vi "Autopatch-v2.2_systemauto.vi"() -> ()   [LabVIEW 2018]
uses:
  <vilib>/userdefined/High Color/IMAQdx.ctl
  <vilib>/DAQmx/write.llb/DAQmx Write (Analog DBL 1Chan 1Samp).vi
  <vilib>/DAQmx/write.llb/DAQmx Write (Analog Wfm 1Chan NSamp).vi
  <vilib>/DAQmx/read.llb/DAQmx Read (Analog Wfm 1Chan NSamp).vi
  <vilib>/Analysis/baseanly.llb/Mean (DBL).vi
  <vilib>/DAQmx/create/channels.llb/DAQmx Create Channel (AO-Voltage-Basic).vi
  <vilib>/DAQmx/miscellaneous.llb/DAQmx Fill In Error Info.vi
  <vilib>/DAQmx/create/channels.llb/DAQmx Create Channel (AI-Voltage-Basic).vi
  <vilib>/DAQmx/configure/timing.llb/DAQmx Timing (Sample Clock).vi
  <vilib>/DAQmx/configure/trigger.llb/DAQmx Start Trigger (Digital Edge).vi
  <vilib>/Waveform/WDTOps.llb/WDT Waveform Duration DBL.vi
  <vilib>/addons/control/pid/pid.llb/PID (DBL).vi
  <vilib>/vision/driver/NI_Vision_Acquisition_Software.lvlib
  <resource>/objmgr/daqmx.rc
  <vilib>/Analysis/NI_AALBase.lvlib
  <vilib>/measure/NI_MABase.lvlib
  <vilib>/vision/NI_Vision_Development_Module.lvlib
  <vilib>/addons/control/pid/NI_PID_pid.lvlib
  <vilib>/Analysis/NI_AALPro.lvlib
panel:
  out "最大值":dbl
  out "Matches 2":T1(array[cluster]) {"Bounding Box"."y" format="%.2f"; "Bounding Box"."x" format="%.2f"; "Position"."y" format="%.2f"; "Position"."x" format="%.2f"; "Score" format="%.2f"; "Scale" format="%.2f"; "Angle" format="%.2f"}
  in  "基路径40":path=path "D:/韩宇/程序/CCD/模板40倍.jpg"
  out "Particle Measurements (Pixels) 2":dbl[][](array[numeric]) format="%.2f"
  in  "Pixel Measurements 2":T2[](array[typedef])=[2] items=["Center of Mass X", "Center of Mass Y", "First Pixel X", "First Pixel Y", "Bounding Rect Left", "Bounding Rect Top", "Bounding Rect Right", "Bounding Rect Bottom", "Max Feret Diameter Start X", "Max Feret Diameter Start Y", "Max Feret Diameter End X", "Max Feret Diameter End Y", "Max Horiz. Segment Length Left", "Max Horiz. Segment Length Right", "Max Horiz. Segment Length Row", "-", "Bounding Rect Width", "Bounding Rect Height", "Bounding Rect Diagonal", "Perimeter", "Convex Hull Perimeter", "Holes' Perimeter", "Max Feret Diameter", "Equivalent Ellipse Major Axis", "Equivalent Ellipse Minor Axis", "Equivalent Ellipse Minor Axis (Feret)", "Equivalent Rect Long Side", "Equivalent Rect Short Side", "Equivalent Rect Diagonal", "Equivalent Rect Short Side (Feret)", "Average Horiz. Segment Length", "Average Vert. Segment Length", "Hydraulic Radius", "Waddel Disk Diameter", "-", "Area", "Holes' Area", "Particle & Holes' Area", "Convex Hull Area", "Image Area", "-", "Number of Holes", "Number of Horiz. Segments", "Number of Vert. Segments", "-", "Orientation", "Max Feret Diameter Orientation", "-", "% Area/Image Area", "% Area/(Particle & Holes' Area)", "Ratio of Equivalent Ellipse Axes", "Ratio of Equivalent Rect Sides", "-", "Elongation Factor", "Compactness Factor", "Heywood Circularity Factor", "Type Factor", "-", "Sum X", "Sum Y", "Sum XX", "Sum XY", "Sum YY", "Sum XXX", "Sum XXY", "Sum XYY", "Sum YYY", "-", "Moment of Inertia XX", "Moment of Inertia XY", "Moment of Inertia YY", "Moment of Inertia XXX", "Moment of Inertia XXY", "Moment of Inertia XYY", "Moment of Inertia YYY", "Norm. Moment of Inertia XX", "Norm. Moment of Inertia XY", "Norm. Moment of Inertia YY", "Norm. Moment of Inertia XXX", "Norm. Moment of Inertia XXY", "Norm. Moment of Inertia XYY", "Norm. Moment of Inertia YYY", "Hu Moment 1", "Hu Moment 2", "Hu Moment 3", "Hu Moment 4", "Hu Moment 5", "Hu Moment 6", "Hu Moment 7"]
  out "傅里叶最大值":dbl
  out "傅里叶数组":bool[](array[boolean])
  in  "傅里叶状态机":u16(ring) items=["傅里叶初始", "傅里叶循环", "傅里叶暂停", "傅里叶结束"]
  out "图像检测到":bool=TRUE
  out "自动封接开始时间":u32
  out "针下降次数":i32
  in  "自动测试":bool
  in  "图像网络检测":bool
  out "写入的字节":i32
  out "数据输出 3":string
  out "X 3":i32
  out "Y 3":i32
  out "error IO":errorcluster
  out "裁剪数组":i32[](array[numeric])
  out "Y 2":i32
  out "X 2":i32
  in  "针尖自动移动 2":bool
  in  "升Z轴找针":bool
  out "已发送图像":bool
  in  "傅里叶":bool
  in  "自动对焦状态机":u16(ring) items=["自动对焦初始", "自动对焦循环", "自动对焦结束"]
  in  "自动扫描状态机":u16(ring) items=["自动扫描初始", "自动扫描循环", "自动扫描结束"]
  out "startY":dbl
  in  "手动暂停":bool
  out "Particle Measurements (Pixels)":dbl[][](array[numeric]) format="%.2f"
  in  "Pixel Measurements":T2[](array[typedef])=[3] items=["Center of Mass X", "Center of Mass Y", "First Pixel X", "First Pixel Y", "Bounding Rect Left", "Bounding Rect Top", "Bounding Rect Right", "Bounding Rect Bottom", "Max Feret Diameter Start X", "Max Feret Diameter Start Y", "Max Feret Diameter End X", "Max Feret Diameter End Y", "Max Horiz. Segment Length Left", "Max Horiz. Segment Length Right", "Max Horiz. Segment Length Row", "-", "Bounding Rect Width", "Bounding Rect Height", "Bounding Rect Diagonal", "Perimeter", "Convex Hull Perimeter", "Holes' Perimeter", "Max Feret Diameter", "Equivalent Ellipse Major Axis", "Equivalent Ellipse Minor Axis", "Equivalent Ellipse Minor Axis (Feret)", "Equivalent Rect Long Side", "Equivalent Rect Short Side", "Equivalent Rect Diagonal", "Equivalent Rect Short Side (Feret)", "Average Horiz. Segment Length", "Average Vert. Segment Length", "Hydraulic Radius", "Waddel Disk Diameter", "-", "Area", "Holes' Area", "Particle & Holes' Area", "Convex Hull Area", "Image Area", "-", "Number of Holes", "Number of Horiz. Segments", "Number of Vert. Segments", "-", "Orientation", "Max Feret Diameter Orientation", "-", "% Area/Image Area", "% Area/(Particle & Holes' Area)", "Ratio of Equivalent Ellipse Axes", "Ratio of Equivalent Rect Sides", "-", "Elongation Factor", "Compactness Factor", "Heywood Circularity Factor", "Type Factor", "-", "Sum X", "Sum Y", "Sum XX", "Sum XY", "Sum YY", "Sum XXX", "Sum XXY", "Sum XYY", "Sum YYY", "-", "Moment of Inertia XX", "Moment of Inertia XY", "Moment of Inertia YY", "Moment of Inertia XXX", "Moment of Inertia XXY", "Moment of Inertia XYY", "Moment of Inertia YYY", "Norm. Moment of Inertia XX", "Norm. Moment of Inertia XY", "Norm. Moment of Inertia YY", "Norm. Moment of Inertia XXX", "Norm. Moment of Inertia XXY", "Norm. Moment of Inertia XYY", "Norm. Moment of Inertia YYY", "Hu Moment 1", "Hu Moment 2", "Hu Moment 3", "Hu Moment 4", "Hu Moment 5", "Hu Moment 6", "Hu Moment 7"]
  in  "手动换物镜":bool
  out "扫描变量":dbl=10.0
  in  "自动扫描":bool
  in  "自动移至工作位置":bool
  out "Z":dbl
  out "Y":dbl
  out "X":dbl
  out "自动接触初始":i32
  in  "枚举":enum16{"200ms", "500ms", "1000ms", ""}(ring)
  out "dX/dt":dbl[](array[numeric])
  in  "下降/向右":bool
  in  "down":bool
  in  "up":bool
  out "Z轴坐标":string
  in  "调焦步伐/um":i64(ring)=3 items=["1", "10", "100", "1000", "10000"]
  in  "停止运动":bool
  in  "设置移动步长":bool
  in  "返回Z轴坐标":bool
  out "x*y":dbl
  out "电阻值":dbl
  in  "钳制电位":i16(ring) items=["0mv", "-70mv"]
  out "起始破膜时间":u32
  in  "自动破膜":bool
  in  "控制箱刺激ON\n/放大器刺激":bool=TRUE
  in  "自动封接":bool
  in  "保存数据":bool
  out "是否匹配到？":bool
  in  "PID gains":T3={"proportional gain (Kc)"=-0.05, "integral time (Ti, min)"=0.0, "derivative time (Td, min)"=0.0} caption="PID增益" {"derivative time (Td, min)" format="%.3f"; "integral time (Ti, min)" format="%.3f"; "proportional gain (Kc)" format="%.3f"}
  in  "PID gains 2":T3={"proportional gain (Kc)"=0.05, "integral time (Ti, min)"=0.0, "derivative time (Td, min)"=0.0} caption="PID增益" {"derivative time (Td, min)" format="%.3f"; "integral time (Ti, min)" format="%.3f"; "proportional gain (Kc)" format="%.3f"}
  out "x+y 2":i16
  out "调焦值2":dbl
  out "调焦值3":dbl
  out "调焦值4":dbl
  out "对焦变量":dbl
  in  "聚焦值数组":dbl[](array[numeric])
  in  "下降步伐/um":dbl=1.0
  in  "自动接触":bool
  out "清晰度评价函数":dbl(graph)
  in  "针尖自动移动":bool
  in  "针尖细对焦":bool
  in  "针尖粗对焦":bool
  out "二值化":T4(plugin-control)
  in  "Range":cluster{"Lower value":sgl, "Upper value":sgl}={"Lower value"=0.0, "Upper value"=157.0} {"Upper value" format="%.2f"; "Lower value" format="%.2f"}
  in  "Operation":T5(ring)=enum."Dilate"
  in  "Number of Erosion":i32=10
  out "Right":dbl
  out "目标坐标":i32[](array[numeric])
  in  "针尖模板匹配":bool=TRUE
  in  "基路径20":path=path "D:/韩宇/程序/CCD/针尖水下模板20X.jpg"
  out "Number of Matches":i32
  in  "Minimum Contrast":i32 min=0 max=255 step=1
  in  "Minimum Match Score":sgl=650.0 min=0 max=1000 format="%.2f"
  in  "Number of Matches Requested":i32=1 min=1
  in  "Match Mode":u16(ring) items=["Shift Invariant", "Rotation Invariant"]
  out "针尖坐标":sgl[](array[numeric])
  in  "入液阻值校准":bool
  out "校准的入液阻值":dbl
  out "错误输出 3":errorcluster caption="错误输出"
  in  "低负开关":bool
  in  "低正开关":bool
  in  "大气压":bool
  in  "高负开关":bool
  in  "高正开关":bool
  in  "case":dbl
  out "测量值":dbl
  out "给定值":dbl
  out "输出气压波形图表":cluster{dbl, "低负":dbl}(graph)
  in  "低负":sgl(knob)=-0.45548448
  in  "高负":sgl(knob)=-5.0
  in  "低正":sgl(knob)=0.49642125 scale=0.0..2.0
  in  "高正":sgl(knob)=10.718505 scale=0.0..15.0
  in  "采样率":u32=255
  in  "DevIndex":i32
  in  "Holding Voltage":dbl=-70.0
  out "Negative Peak":dbl
  out "阻值波形图表":dbl(graph)
  out "Resistance(MΩ)":dbl
  out "！":bool
  in  "电压钳/电流钳":u16(ring) items=["Voltage Clamp", "Current Clamp"]
  out "电流信号波形图":waveform(dbl)(graph)
  in  "frequency":dbl=20.0
  in  "Averaging":i32=5
  in  "amplitude":dbl=0.01
  in  "阻值数组":dbl[](array[numeric])
  out "循环时间":u32
  out "Image":T4(plugin-control)
  out "错误输出":errorcluster
  in  "停止":bool
  in  "Session In":T6="cam1"
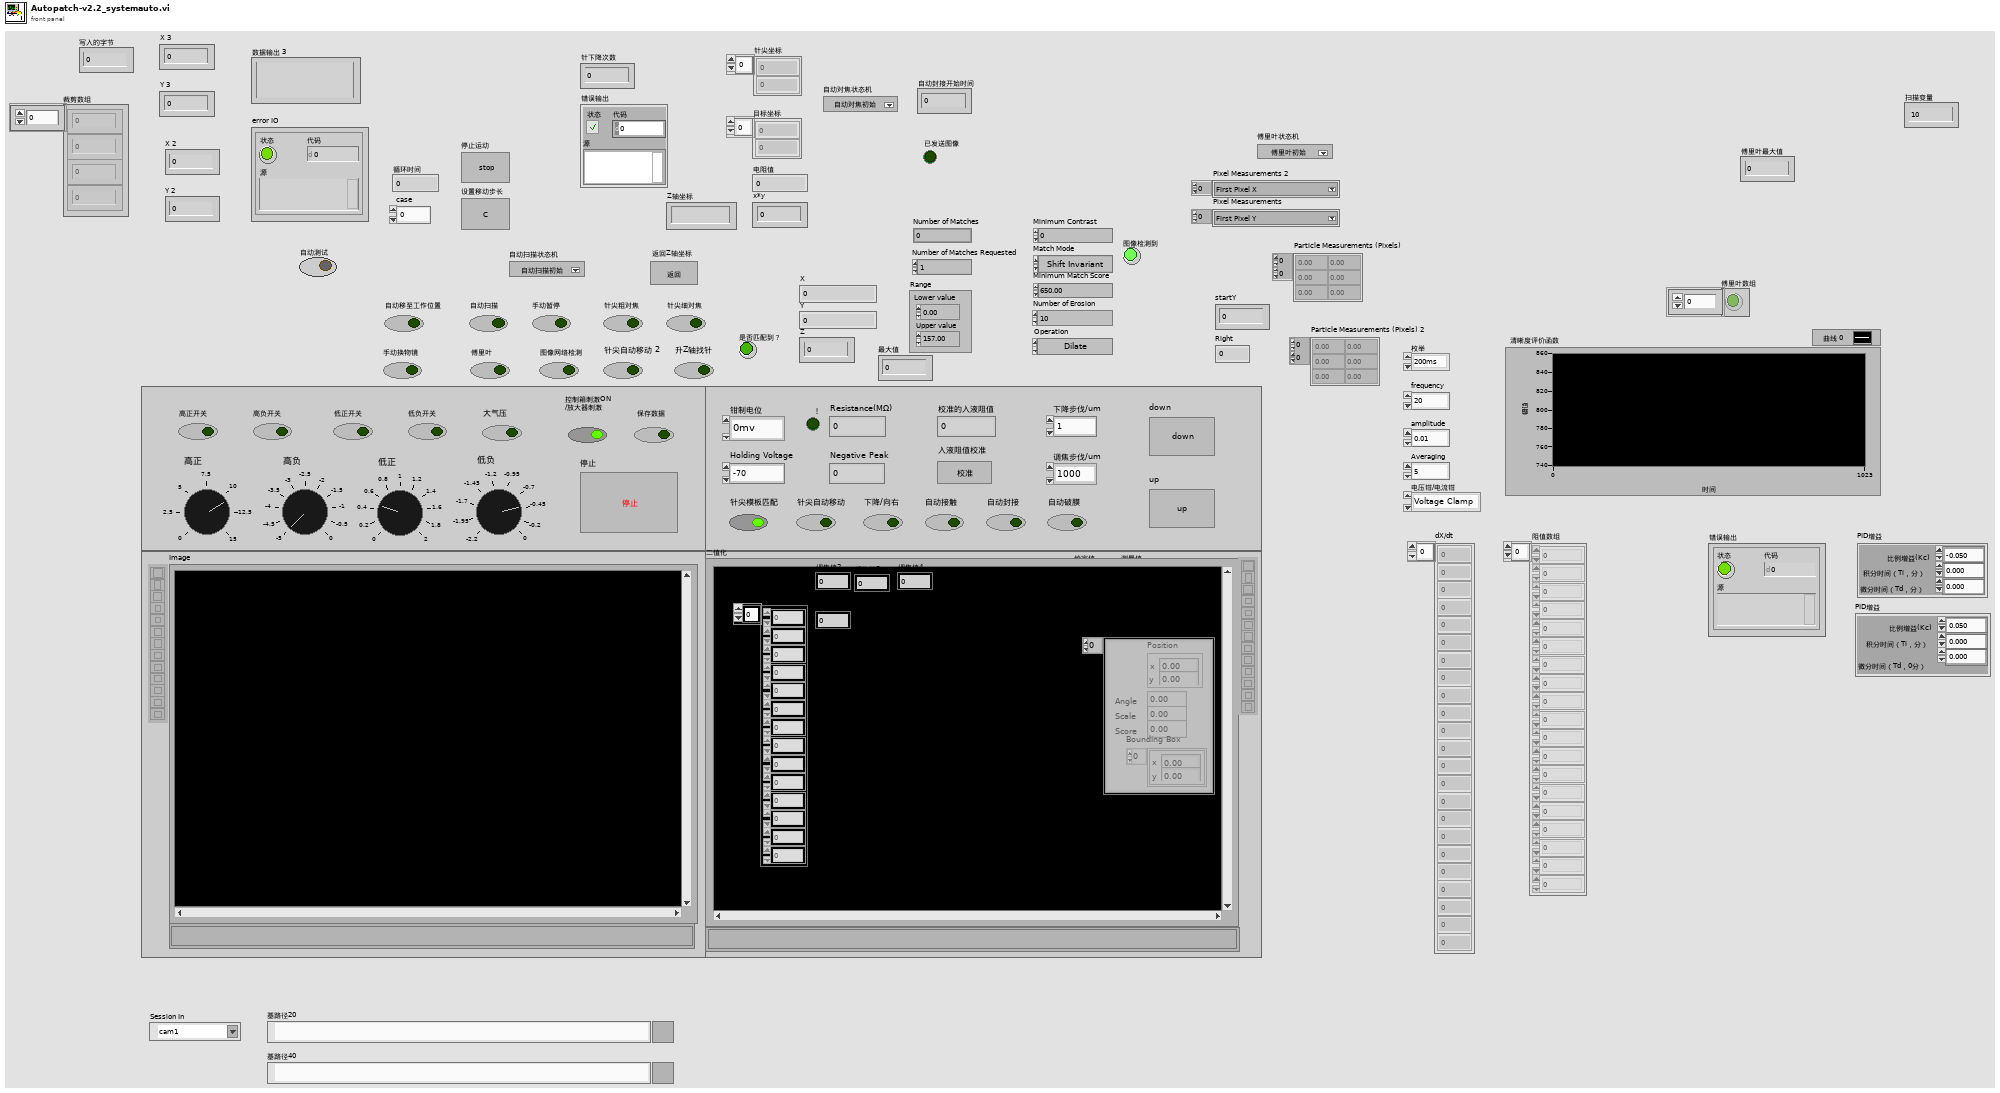
[diagram p1: front panel]
types:
  T1 = cluster{"Position":cluster{"x":sgl, "y":sgl}, "Angle":sgl, "Scale":sgl, "Score":sgl, "Bounding Box":cluster{"x":sgl, "y":sgl}[]}[]
  T2 = typedef "Particle Parameters" = i32
  T3 = cluster{"proportional gain (Kc)":dbl, "integral time (Ti, min)":dbl, "derivative time (Td, min)":dbl}
  T4 = typedef "IMAQ Image.ctl" = refnum<image>
  T5 = enum32{"AutoM", "Close", "Dilate", "Erode", "Gradient", "Gradient out", "Gradient in", "Hit miss", "Open", "PClose", "POpen", "Thick", "Thin"}
  T6 = typedef "IMAQdx.ctl" = refnum<k21>
  T7 = typedef "Image Type" = u32
  T8 = enum16{"open", "replace", "create", "open or create", "replace or create", "replace or create with confirmation"}
  T9 = cluster{"Averaging":i32, "frequency":dbl, "amplitude":dbl, "Proportion":dbl, "Fs":dbl}
  T10 = enum16{"Sine Wave", "Triangle Wave", "Square Wave", "Sawtooth Wave"}
  T11 = cluster{"Global Rectangle":i32[], "Contours":cluster{"Contour Type":u32, "ROI Type":u32, "Points":i32[]}[]}
  T12 = cluster{"Position":cluster{"x":sgl, "y":sgl}, "Angle":sgl, "Scale":sgl, "Score":sgl, "Bounding Box":cluster{"x":sgl, "y":sgl}[]}
  T13 = enum32{"Real", "Imaginary", "Magnitude", "Phase"}
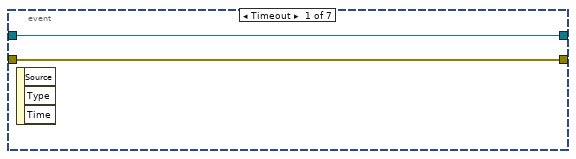
[diagram p3: hidden frame]
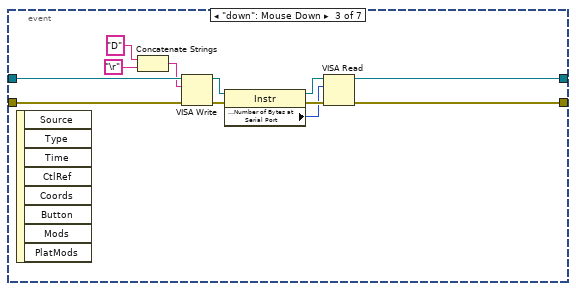
[diagram p4: hidden frame]
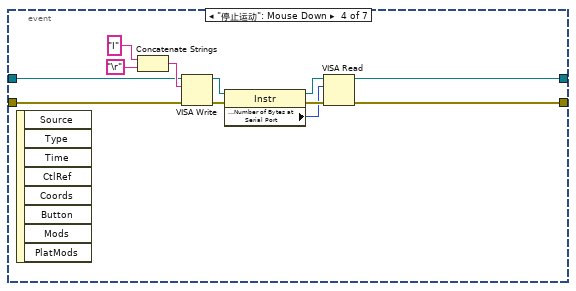
[diagram p5: hidden frame]
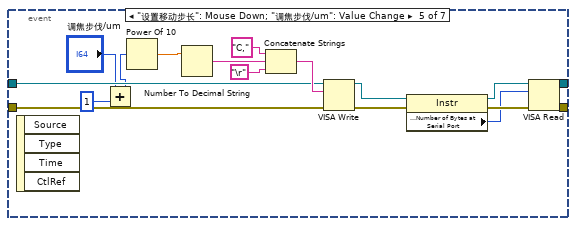
[diagram p6: hidden frame]
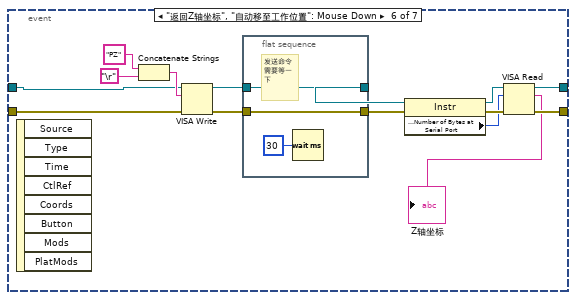
[diagram p7: hidden frame]
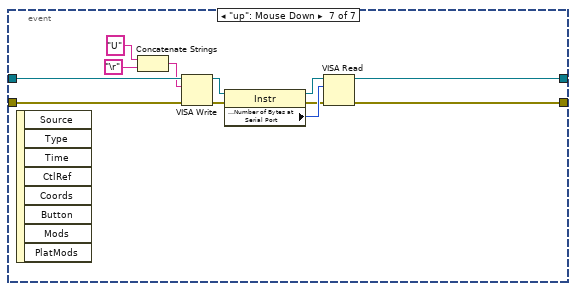
[diagram p8: hidden frame]
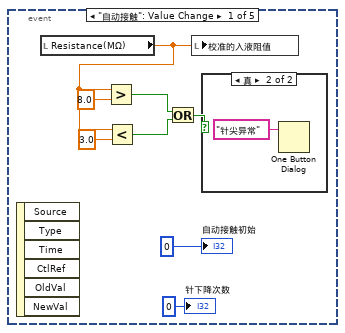
[diagram p9: hidden frame]
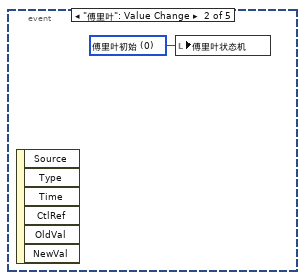
[diagram p11: hidden frame]
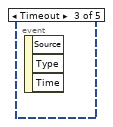
[diagram p12: hidden frame]
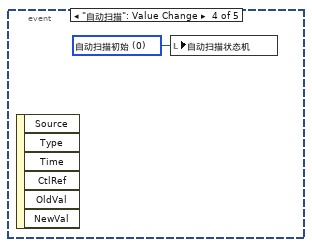
[diagram p13: hidden frame]
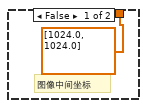
[diagram p14: hidden frame]
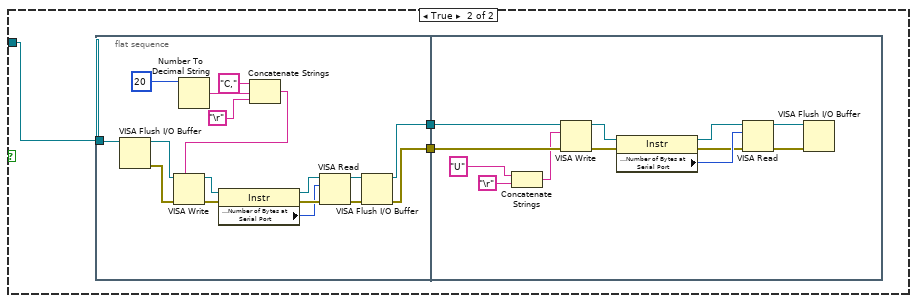
[diagram p16: hidden frame]
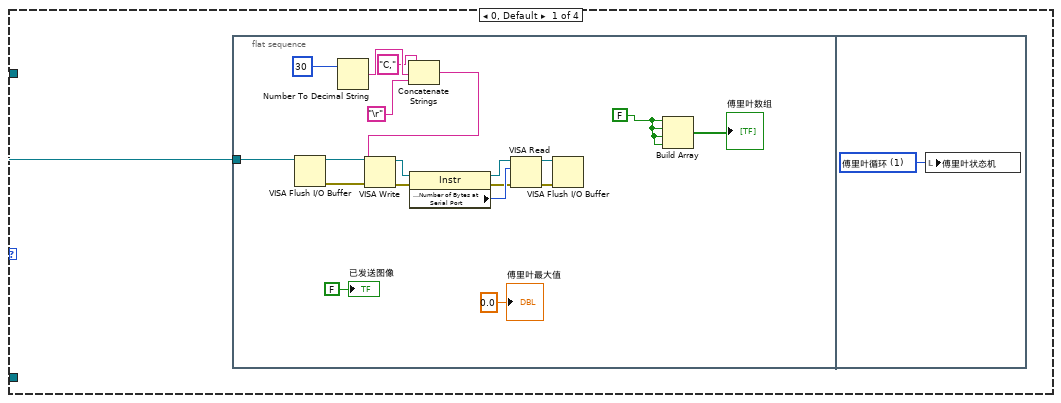
[diagram p18: hidden frame]
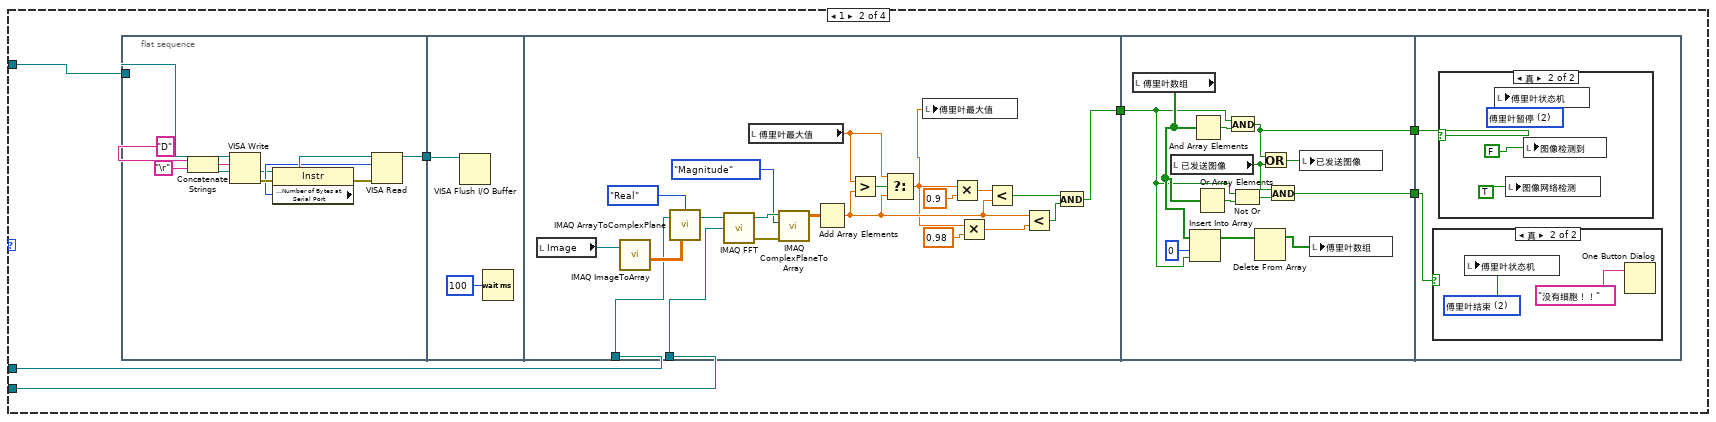
[diagram p19: hidden frame]
diagram:
  w5 = T7 0 items=["Grayscale (U8)", "Grayscale (I16)", "Grayscale (SGL)", "Complex (CSG)", "RGB (U32)", "HSL (U32)", "RGB (U64)", "Grayscale (U16)"] ("Image Type")
  w16 = T7 3 items=["Grayscale (U8)", "Grayscale (I16)", "Grayscale (SGL)", "Complex (CSG)", "RGB (U32)", "HSL (U32)", "RGB (U64)", "Grayscale (U16)"] ("Image Type")
  w14 = T7 3 items=["Grayscale (U8)", "Grayscale (I16)", "Grayscale (SGL)", "Complex (CSG)", "RGB (U32)", "HSL (U32)", "RGB (U64)", "Grayscale (U16)"] ("Image Type")
  w68 = T7 0 items=["Grayscale (U8)", "Grayscale (I16)", "Grayscale (SGL)", "Complex (CSG)", "RGB (U32)", "HSL (U32)", "RGB (U64)", "Grayscale (U16)"] ("Image Type")
  w82 = FALSE
  # "XY移动平台"
  # "Mp285"
  # "保存数据"
  n1 = case shown="真" "自动测试" {
    frame False {
    }
    frame True {
      n2 = flat-sequence {
        frame #0 {
          n3 = One Button Dialog(message="请安装玻璃电极并手动更换20倍显微镜" ("消息")) -> ()  [unwired: 1 in, 1 out]
        }
        frame #1 {
          n4 = local write "针尖粗对焦"(FALSE ("针尖粗对焦")) -> ()
          n5 = local write "针尖细对焦"(FALSE ("针尖细对焦")) -> ()
          n6 = local write "自动移至工作位置"(TRUE ("自动移至工作位置")) -> ()
          n7 = local write "傅里叶"(FALSE ("傅里叶")) -> ()
          n8 = local write "针尖自动移动"(FALSE ("针尖自动移动")) -> ()
          n9 = local write "针尖自动移动 2"(FALSE ("针尖自动移动 2")) -> ()
          n10 = local write "自动扫描"(FALSE ("自动扫描")) -> ()
          n11 = local write "手动换物镜"(FALSE ("手动换物镜")) -> ()
          n12 = local write "自动接触"(FALSE ("自动接触")) -> ()
          n13 = local write "升Z轴找针"(FALSE ("升Z轴找针")) -> ()
        }
      }
    }
  }
  n14 = flat-sequence {
    tunnel: [w156] -> w129
    frame #0 {
      # "选择刺激方式，内部刺激更准"
      n15 = Array Size(array="阻值数组") -> (size(s)=w155:i32)
      n16 = Delete From Array(array="阻值数组", length=w155) -> (array with subset deleted=w153:dbl[])  [unwired: 1 in, 1 out]
      n17 = local write "阻值数组"(w153) -> ()
    }
    frame #1 {
      # "波形个数"
      # "计算电阻波形比例"
      n18 = Bundle("Averaging"="Averaging", "frequency"="frequency", "amplitude"="amplitude", "Proportion"=0.4, "Fs"=20000.0) -> (w156:T9)  [unwired: 1 in]
    }
  }
  n19 = call "OpenDevice.vi"("DevIndex"="DevIndex") -> ("错误输出"=w109:errorcluster, "DevIndex Output"=w107:i32)  [unwired: 9 in]
  n20 = call "SetUSB2AiRange.vi"("错误输入（无错误）"=w109, "Range"=sgl 5.0, "DevIndex"=w107) -> ("错误输出"=w118:errorcluster, "DevIndex Output"=w116:i32)  [unwired: 7 in]
  n21 = call <vilib>:"IMAQdx Open Camera.vi"("Session In"="Session In") -> ("error out"=w141:errorcluster, "Session Out"=w138:T6)  [unwired: 9 in]
  n22 = call "IMAQ Create"("Image Name"="针尖模板40倍", "Image Type"=w5) -> ("New Image"=w4:T4)  [unwired: 3 in, 1 out]
  n23 = Obtain Queue(element data type=FALSE) -> (queue out=w27:refnum<queue>, error out=w26:errorcluster)  [unwired: 4 in, 1 out]
  n24 = call "IMAQ Create"("Image Name"="针尖模板20倍", "Image Type"=w68) -> ("New Image"=w69:T4)  [unwired: 3 in, 1 out]
  n25 = call "SetSampleRate.vi"("错误输入（无错误）"=w118, "SampleRate"="采样率", "DevIndex"=w116) -> ("错误输出"=w119:errorcluster, "DevIndex Output"=w117:i32)  [unwired: 7 in]
  n26 = call "IMAQ ReadFile 2"("File Path"="基路径40", "Image"=w4) -> ("Image Out"=w2:T4)  [unwired: 5 in, 4 out]
  n27 = call "IMAQ ReadFile 2"("File Path"="基路径20", "Image"=w69) -> ("Image Out"=w67:T4)  [unwired: 5 in, 4 out]
  n28 = call <vilib>:"IMAQdx Configure Grab.vi"("error in"=w141, "Session In"=w138) -> ("error out"=w126:errorcluster, "Session Out"=w139:T6)  [unwired: 8 in]
  n29 = call "SetTrigSource.vi"("错误输入（无错误）"=w119, "TrigSource"=u8 0, "DevIndex"=w117) -> ("错误输出"=w114:errorcluster, "DevIndex Output"=w113:i32)  [unwired: 7 in]
  n30 = call "IMAQ Create"("Image Name"="原图像") -> ("New Image"=w137:T4, "error out"=w124:errorcluster)  [unwired: 4 in]
  n31 = call "IMAQ Create"("Image Name"="灰度图") -> ("New Image"=w130:T4)  [unwired: 4 in, 1 out]
  n32 = call "SetSoftTrig.vi"("错误输入（无错误）"=w114, "Trig"=u8 1, "DevIndex"=w113) -> ("错误输出"=w110:errorcluster, "DevIndex Output"=w108:i32)  [unwired: 7 in]
  n33 = call "285_Initialize.vi"() -> ("VISA资源名称输出"=w25:refnum<visa-resource-name>)  [unwired: 10 in, 1 out]
  n34 = call "285_Initialize_1.vi"() -> ("VISA资源名称输出"=w24:refnum<visa-resource-name>)  [unwired: 10 in, 1 out]
  n35 = call "InitDA.vi"("错误输入（无错误）"=w110, "DevIndex"=w108) -> ("错误输出"=w104:errorcluster, "DevIndex Output"=w105:i32)  [unwired: 8 in]
  n36 = call "PRIOR_Initialize.vi"() -> ("错误输出"=w23:errorcluster, "VISA资源名称输出"=w19:refnum<visa-resource-name>)  [unwired: 10 in]
  n37 = while {
    tunnel: w19 -> [w171]
    tunnel: [w168] -> w28
    tunnel: [w172] -> w29
    tunnel: w27 -> [w165]
    tunnel: w26 -> [w164]
    tunnel: w23 -> [w162]
    stop <- w163 stop-if-true
    n38 = VISA Flush I/O Buffer(VISA resource name=w171, error in (no error)=w162) -> (VISA resource name out=w170:refnum<visa-resource-name>, error out=w169:errorcluster)  [unwired: 1 in]
    n39 = Dequeue Element(queue=w165, timeout in ms (-1)=1 ("超时毫秒(-1)"), error in (no error)=w164) -> (error out=w167:errorcluster)  [unwired: 3 out]
    n40 = event shown="[1] \"up\", \"down\": 鼠标释放" {
      selector: _ -> [_ _ _ _ _ _ _]
      dyn-events: _ -> [_ _ _ _ _ _ _]
      timeout: 1 -> [_ _ _ _ _ _ _]
      tunnel: [w175 w177 w199 w201 w219 w235 w258] -> w172
      tunnel: [w174 w176 w198 w200 w218 w234 w257] -> w168
      tunnel: w170 -> [w175 w179 w197 w203 w221 w237 w256]
      tunnel: w169 -> [w174 w178 w196 w202 w220 w236 w255]
      event Timeout {
        n41 = event-data() -> ()  [unwired: 1 in, 3 out]
      }
      event "up", "down": Mouse Up {
        n42 = event-data() -> ()  [unwired: 1 in, 8 out]
        n43 = Concatenate Strings("I" ("写入缓冲区"), "\r") -> (w187:string)
        n44 = VISA Write ("VISA写入")(VISA resource name=w179, write buffer=w187, error in (no error)=w178) -> (VISA resource name out=w181:refnum<visa-resource-name>, error out=w180:errorcluster)  [unwired: 1 out]
        n45 = property class="Instr"(reference=w181, error in=w180) -> (reference out=w182:refnum<visa-resource-name>, error out=w183:errorcluster, "Serial Settings:Number of Bytes at Serial Port"=w184:u32)
        n46 = VISA Read(VISA resource name=w182, byte count=w184, error in (no error)=w183) -> (VISA resource name out=w177:refnum<visa-resource-name>, error out=w176:errorcluster)  [unwired: 2 out]
      }
      event "down": Mouse Down {
        n47 = event-data() -> ()  [unwired: 1 in, 8 out]
        n48 = Concatenate Strings("D" ("写入缓冲区"), "\r") -> (w188:string)
        n49 = VISA Write ("VISA写入")(VISA resource name=w197, write buffer=w188, error in (no error)=w196) -> (VISA resource name out=w194:refnum<visa-resource-name>, error out=w195:errorcluster)  [unwired: 1 out]
        n50 = property class="Instr"(reference=w194, error in=w195) -> (reference out=w193:refnum<visa-resource-name>, error out=w192:errorcluster, "Serial Settings:Number of Bytes at Serial Port"=w191:u32)
        n51 = VISA Read(VISA resource name=w193, byte count=w191, error in (no error)=w192) -> (VISA resource name out=w199:refnum<visa-resource-name>, error out=w198:errorcluster)  [unwired: 2 out]
      }
      event "停止运动": Mouse Down {
        n52 = event-data() -> ()  [unwired: 1 in, 8 out]
        n53 = Concatenate Strings("I" ("写入缓冲区"), "\r") -> (w204:string)
        n54 = VISA Write ("VISA写入")(VISA resource name=w203, write buffer=w204, error in (no error)=w202) -> (VISA resource name out=w210:refnum<visa-resource-name>, error out=w211:errorcluster)  [unwired: 1 out]
        n55 = property class="Instr"(reference=w210, error in=w211) -> (reference out=w209:refnum<visa-resource-name>, error out=w208:errorcluster, "Serial Settings:Number of Bytes at Serial Port"=w207:u32)
        n56 = VISA Read(VISA resource name=w209, byte count=w207, error in (no error)=w208) -> (VISA resource name out=w201:refnum<visa-resource-name>, error out=w200:errorcluster)  [unwired: 2 out]
      }
      event "设置移动步长": Mouse Down; "调焦步伐/um": Value Change {
        n57 = event-data() -> ()  [unwired: 1 in, 4 out]
        n58 = Add(x="调焦步伐/um", y=i64 1) -> (x+y=w212:i64)
        n59 = Power Of 10(x=w212) -> (10^x=w215:dbl)
        n60 = Number To Decimal String(number=w215) -> (decimal integer string=w216:string)  [unwired: 1 in]
        n61 = Concatenate Strings("C," ("写入缓冲区"), w216, "\r") -> (w222:string)
        n62 = VISA Write ("VISA写入")(VISA resource name=w221, write buffer=w222, error in (no error)=w220) -> (VISA resource name out=w227:refnum<visa-resource-name>, error out=w228:errorcluster)  [unwired: 1 out]
        n63 = property class="Instr"(reference=w227, error in=w228) -> (reference out=w226:refnum<visa-resource-name>, error out=w225:errorcluster, "Serial Settings:Number of Bytes at Serial Port"=w224:u32)
        n64 = VISA Read(VISA resource name=w226, byte count=w224, error in (no error)=w225) -> (VISA resource name out=w219:refnum<visa-resource-name>, error out=w218:errorcluster)  [unwired: 2 out]
      }
      event "返回Z轴坐标", "自动移至工作位置": Mouse Down {
        n65 = event-data() -> ()  [unwired: 1 in, 8 out]
        n66 = Concatenate Strings("PZ" ("写入缓冲区"), "\r") -> (w239:string)
        n67 = VISA Write ("VISA写入")(VISA resource name=w237, write buffer=w239, error in (no error)=w236) -> (VISA resource name out=w233:refnum<visa-resource-name>, error out=w232:errorcluster)  [unwired: 1 out]
        n68 = flat-sequence {
          tunnel: w233 -> [w245]
          tunnel: w232 -> [w246]
          tunnel: [w246] -> w230
          tunnel: [w245] -> w231
          frame #0 {
            # "发送命令需要等一下"
            n69 = Wait (ms)(milliseconds to wait=u32 30 ("等待时间（毫秒）")) -> ()  [unwired: 1 out]
          }
        }
        n70 = property class="Instr"(reference=w231, error in=w230) -> (reference out=w243:refnum<visa-resource-name>, error out=w242:errorcluster, "Serial Settings:Number of Bytes at Serial Port"=w241:u32)
        n71 = VISA Read(VISA resource name=w243, byte count=w241, error in (no error)=w242) -> (VISA resource name out=w235:refnum<visa-resource-name>, read buffer=→"Z轴坐标":string, error out=w234:errorcluster)  [unwired: 1 out]
      }
      event "up": Mouse Down {
        n72 = event-data() -> ()  [unwired: 1 in, 8 out]
        n73 = Concatenate Strings("U" ("写入缓冲区"), "\r") -> (w252:string)
        n74 = VISA Write ("VISA写入")(VISA resource name=w256, write buffer=w252, error in (no error)=w255) -> (VISA resource name out=w251:refnum<visa-resource-name>, error out=w250:errorcluster)  [unwired: 1 out]
        n75 = property class="Instr"(reference=w251, error in=w250) -> (reference out=w248:refnum<visa-resource-name>, error out=w247:errorcluster, "Serial Settings:Number of Bytes at Serial Port"=w249:u32)
        n76 = VISA Read(VISA resource name=w248, byte count=w249, error in (no error)=w247) -> (VISA resource name out=w258:refnum<visa-resource-name>, error out=w257:errorcluster)  [unwired: 2 out]
      }
    }
    n77 = Unbundle By Name(w167) -> ("status"=w163:bool)
  }
  n78 = while {
    tunnel: w105 -> [w271]
    tunnel: w27 -> [w310]
    tunnel: w26 -> [w309]
    tunnel: [w263] -> w31
    tunnel: w104 -> [w270]
    tunnel: [w261] -> w30
    stop <- w306 stop-if-true
    # "气压控制循环"
    # "气压到电压转换"
    n79 = Dequeue Element(queue=w310, timeout in ms (-1)=1 ("超时毫秒(-1)"), error in (no error)=w309) -> (error out=w307:errorcluster)  [unwired: 3 out]
    n80 = Unbundle By Name(w307) -> ("status"=w306:bool)
    n81 = In Range and Coerce(upper limit=sgl 15.0 ("上限"), x="高正", lower limit=sgl 0.0 ("下限")) -> (coerced(x)=w274:sgl)  [unwired: 1 out]
    n82 = In Range and Coerce(upper limit=sgl 0.0 ("上限"), x="高负", lower limit=sgl -5.0 ("下限")) -> (coerced(x)=w278:sgl)  [unwired: 1 out]
    n83 = Divide(x=w274, y=3) -> (x/y=w295:sgl)
    n84 = Divide(x=w278, y=-1.004) -> (x/y=w291:dbl)
    n85 = In Range and Coerce(upper limit=sgl 2.0 ("上限"), x="低正", lower limit=sgl 0.0 ("下限")) -> (coerced(x)=w282:sgl)  [unwired: 1 out]
    n86 = call "SetDA.vi"("错误输入（无错误）"=w270, "DAVolt"=w295, "DANum"=u8 0, "DevIndex"=w271) -> ("错误输出"=w304:errorcluster, "DevIndex Output"=w305:i32)  [unwired: 6 in]
    n87 = In Range and Coerce(upper limit=sgl 0.0 ("上限"), x="低负", lower limit=sgl -2.2 ("下限")) -> (coerced(x)=w284:sgl)  [unwired: 1 out]
    n88 = call "SetDA.vi"("错误输入（无错误）"=w304, "DAVolt"=w291, "DANum"=u8 1, "DevIndex"=w305) -> ("错误输出"=w303:errorcluster, "DevIndex Output"=w302:i32)  [unwired: 6 in]
    n89 = Multiply(x=w282, y=2.564) -> (x*y=w288:dbl)
    n90 = Multiply(x=w284, y=-2.294) -> (x*y=w289:dbl)
    n91 = call "SetDA.vi"("错误输入（无错误）"=w303, "DAVolt"=w288, "DANum"=u8 2, "DevIndex"=w302) -> ("错误输出"=w300:errorcluster, "DevIndex Output"=w301:i32)  [unwired: 6 in]
    n92 = call "SetDA.vi"("错误输入（无错误）"=w300, "DAVolt"=w289, "DANum"=u8 3, "DevIndex"=w301) -> ("错误输出"=w264:errorcluster, "DevIndex Output"=w265:i32)  [unwired: 6 in]
    n93 = event shown="[4] \"低负开关\": 值改变" {
      selector: _ -> [_ _ _ _ _ _ _ _]
      dyn-events: _ -> [_ _ _ _ _ _ _ _]
      timeout: 1 -> [_ _ _ _ _ _ _ _]
      event "高正开关": Value Change {
        n94 = event-data() -> ("OldVal"=w389:bool)  [unwired: 1 in, 5 out]
        n95 = local read "高正开关"() -> (w390:bool)
        n96 = case shown="真" w390 {
          tunnel: w389 -> [_ w392]
          frame False {
          }
          frame True {
            n97 = local write "高负开关"(w392) -> ()
            n98 = local write "低负开关"(w392) -> ()
            n99 = local write "低正开关"(w392) -> ()
            n100 = local write "大气压"(w392) -> ()
            n101 = local write "case"(1.0) -> ()
          }
        }
      }
      event Timeout {
        n102 = event-data() -> ()  [unwired: 1 in, 3 out]
      }
      event "大气压": Value Change {
        n103 = event-data() -> ("OldVal"=w393:bool)  [unwired: 1 in, 5 out]
        n104 = local read "大气压"() -> (w394:bool)
        n105 = case shown="真" w394 {
          tunnel: w393 -> [_ w396]
          frame False {
          }
          frame True {
            n106 = local write "高负开关"(w396) -> ()
            n107 = local write "低正开关"(w396) -> ()
            n108 = local write "低负开关"(w396) -> ()
            n109 = local write "高正开关"(w396) -> ()
            n110 = local write "case"(5.0) -> ()
          }
        }
      }
      event "低正开关": Value Change {
        n111 = event-data() -> ("OldVal"=w398:bool)  [unwired: 1 in, 5 out]
        n112 = local read "低正开关"() -> (w397:bool)
        n113 = case shown="真" w397 {
          tunnel: w398 -> [_ w400]
          frame False {
          }
          frame True {
            n114 = local write "高正开关"(w400) -> ()
            n115 = local write "高负开关"(w400) -> ()
            n116 = local write "低负开关"(w400) -> ()
            n117 = local write "大气压"(w400) -> ()
            n118 = local write "case"(3.0) -> ()
          }
        }
      }
      event "低负开关": Value Change {
        n119 = event-data() -> ("OldVal"=w402:bool)  [unwired: 1 in, 5 out]
        n120 = local read "低负开关"() -> (w401:bool)
        n121 = case shown="真" w401 {
          tunnel: w402 -> [_ w404]
          frame False {
          }
          frame True {
            n122 = local write "高负开关"(w404) -> ()
            n123 = local write "低正开关"(w404) -> ()
            n124 = local write "高正开关"(w404) -> ()
            n125 = local write "大气压"(w404) -> ()
            n126 = local write "case"(4.0) -> ()
          }
        }
      }
      event "高负开关": Value Change {
        n127 = event-data() -> ("OldVal"=w406:bool)  [unwired: 1 in, 5 out]
        n128 = local read "高负开关"() -> (w405:bool)
        n129 = case shown="真" w405 {
          tunnel: w406 -> [_ w408]
          frame False {
          }
          frame True {
            n130 = local write "低正开关"(w408) -> ()
            n131 = local write "低负开关"(w408) -> ()
            n132 = local write "高正开关"(w408) -> ()
            n133 = local write "大气压"(w408) -> ()
            n134 = local write "case"(2.0) -> ()
          }
        }
      }
      event "自动封接": Value Change {
        # "初始值"
        n135 = event-data() -> ()  [unwired: 1 in, 6 out]
        n136 = Tick Count (ms)() -> (millisecond timer value=→"自动封接开始时间":u32)
        n137 = local write "低负"(-0.66) -> ()
      }
      event "自动破膜": Value Change {
        n138 = event-data() -> ()  [unwired: 1 in, 6 out]
        n139 = Tick Count (ms)() -> (millisecond timer value=→"起始破膜时间":u32)
      }
    }
    n140 = case shown="真" "自动封接" {
      frame False {
      }
      frame True {
        w349 = 1300.0 ("y")
        # "阈值确定？？"
        # "气压微调"
        n141 = local read "阻值数组"() -> (w350:dbl[])
        n142 = local read "阻值数组"() -> (w348:dbl[])
        n143 = Index Array(array=w350, index=0 ("索引")) -> (element=w352:dbl)
        n144 = Index Array(array=w350, index=1 ("索引")) -> (element=w351:dbl)
        n145 = Index Array(array=w350, index=2 ("索引")) -> (element=w355:dbl)
        n146 = Index Array(array=w350, index=3 ("索引")) -> (element=w354:dbl)
        n147 = Index Array(array=w350, index=4 ("索引")) -> (element=w353:dbl)
        n148 = call <vilib>:"Derivative x(t).vi"("X"=w348) -> ("dX/dt"=w345:dbl[])  [unwired: 9 in, 1 out]
        "dX/dt" <- w345
        n149 = Greater?(x=w352, y=w349) -> (0:w340:bool)
        n150 = Greater?(x=w355, y=w349) -> (0:w338:bool)
        n151 = Greater?(x=w351, y=w349) -> (0:w339:bool)
        n152 = Greater?(x=w354, y=w349) -> (0:w337:bool)
        n153 = Greater?(x=w353, y=w349) -> (0:w336:bool)
        n154 = Index Array(array=w345, index=0 ("索引")) -> (element=w341:dbl)
        n155 = Compound Arithmetic op=AND ("复合运算")(w340, w339, w338, w337, w336) -> (w335:bool)
        n156 = Greater?(x=w341, y=0.0) -> (0:w347:bool)
        n157 = Less?(x=w341, y=0.0) -> (x < y?=w346:bool)
        n158 = case shown="假" w335 {
          frame True {
            n159 = flat-sequence {
              frame #0 {
                w373 = FALSE
                n160 = local write "高负开关"(w373) -> ()
                n161 = local write "低负开关"(w373) -> ()
                n162 = local write "低正开关"(w373) -> ()
                n163 = local write "高正开关"(w373) -> ()
                n164 = local write "大气压"(TRUE) -> ()
              }
              frame #1 {
                n165 = local write "case"(5.0) -> ()
              }
              frame #2 {
                n166 = local write "自动破膜"(TRUE) -> ()
                n167 = local write "自动封接"(FALSE) -> ()
                n168 = One Button Dialog(message="已形成G欧封接！" ("消息")) -> ()  [unwired: 1 in, 1 out]
              }
            }
          }
          frame False {
            n169 = flat-sequence {
              frame #0 {
                w379 = FALSE
                n170 = local write "高负开关"(w379) -> ()
                n171 = local write "低正开关"(w379) -> ()
                n172 = local write "高正开关"(w379) -> ()
                n173 = local write "低负开关"(TRUE) -> ()
                n174 = local write "大气压"(w379) -> ()
              }
              frame #1 {
                n175 = local write "case"(4.0) -> ()
              }
              frame #2 {
                n176 = local read "自动封接开始时间"() -> (w385:u32)
                n177 = Tick Count (ms)() -> (millisecond timer value=w386:u32)
                n178 = Subtract(x=w386, y=w385) -> (x-y=w384:u32)
                n179 = Greater?(x=w384, y=u32 100000) -> (0:w382:bool)
                n180 = case shown="真" w382 {
                  frame False {
                  }
                  frame True {
                    n181 = local write "自动封接"(FALSE) -> ()
                    n182 = One Button Dialog(message="自动封接失败！！" ("消息")) -> ()  [unwired: 1 in, 1 out]
                  }
                }
              }
            }
          }
        }
        n183 = case shown="真" w347 {
          frame False {
          }
          frame True {
            n184 = local read "低负"() -> (w368:sgl)
            n185 = Add(x=-0.05, y=w368) -> (x+y=w371:dbl)
            n186 = In Range and Coerce(upper limit=0.0, x=w371, lower limit=-2.0) -> (coerced(x)=w367:dbl)  [unwired: 1 out]
            n187 = local write "低负"(w367) -> ()
          }
        }
        n188 = case shown="真" w346 {
          frame False {
          }
          frame True {
            n189 = local read "低负"() -> (w362:sgl)
            n190 = Add(x=0.05, y=w362) -> (x+y=w365:dbl)
            n191 = In Range and Coerce(upper limit=0.0, x=w365, lower limit=-2.0) -> (coerced(x)=w361:dbl)  [unwired: 1 out]
            n192 = local write "低负"(w361) -> ()
          }
        }
      }
    }
    n193 = case shown="4" "case" {
      tunnel: w265 -> [w415 w435 w457 w481 w505 w518]
      tunnel: w264 -> [w414 w434 w456 w480 w504 w517]
      tunnel: [w415 w417 w448 w475 w497 w515] -> w263
      tunnel: [w414 w425 w449 w474 w498 w514] -> w261
      tunnel: [w412 w416 w440 w464 w488 w512] -> w267
      frame Default {
        w413 = 0.0
        n194 = Bundle(w413, w413) -> (w412:cluster{dbl, dbl})  [unwired: 1 in]
      }
      frame 1 {
        w432 = TRUE
        w433 = FALSE
        n195 = Build Array(w433, w432, w432, w433, w433, w433, w433, w433) -> (w436:bool[])
        n196 = Boolean Array To Number(Boolean array=w436) -> (number=w439:u32)
        n197 = To Unsigned Byte Integer(number=w439) -> (unsigned 8bit integer=w438:u8)
        n198 = call "StartRead.vi"("错误输入（无错误）"=w434, "DevIndex"=w435) -> ("错误输出"=w430:errorcluster, "DevIndex Output"=w431:i32)  [unwired: 8 in]
        n199 = call "SetDioOut.vi"("错误输入（无错误）"=w430, "DioOut"=w438, "DioChanSel"=u8 255, "DevIndex"=w431) -> ("错误输出"=w426:errorcluster, "DevIndex Output"=w427:i32)  [unwired: 6 in]
        n200 = call "GetAiChans.vi"("错误输入（无错误）"=w426, "Num"=u32 1, "ChanSel"=u16 1, "DevIndex"=w427) -> ("错误输出"=w425:errorcluster, "Ai"=w422:sgl[][], "DevIndex Output"=w417:i32)  [unwired: 4 in, 1 out]
        n201 = Index Array(array=w422, index (row)=0, index (col)=0) -> (element=w419:sgl)
        n202 = local read "高正"() -> (w421:sgl)
        n203 = Multiply(x=w419, y=3) -> (x*y=w418:sgl)
        n204 = Bundle(w418, "高正"=w421) -> (w416:cluster{sgl, "高正":sgl})  [unwired: 1 in]
      }
      frame 2 {
        w455 = TRUE
        w454 = FALSE
        n205 = Build Array(w454, w455, w454, w454, w455, w454, w454, w454) -> (w458:bool[])
        n206 = Boolean Array To Number(Boolean array=w458) -> (number=w463:u32)
        n207 = To Unsigned Byte Integer(number=w463) -> (unsigned 8bit integer=w462:u8)
        n208 = call "StartRead.vi"("错误输入（无错误）"=w456, "DevIndex"=w457) -> ("错误输出"=w459:errorcluster, "DevIndex Output"=w460:i32)  [unwired: 8 in]
        n209 = call "SetDioOut.vi"("错误输入（无错误）"=w459, "DioOut"=w462, "DioChanSel"=u8 255, "DevIndex"=w460) -> ("错误输出"=w450:errorcluster, "DevIndex Output"=w451:i32)  [unwired: 6 in]
        n210 = call "GetAiChans.vi"("错误输入（无错误）"=w450, "Num"=u32 1, "ChanSel"=u16 2, "DevIndex"=w451) -> ("错误输出"=w449:errorcluster, "Ai"=w445:sgl[][], "DevIndex Output"=w448:i32)  [unwired: 4 in, 1 out]
        n211 = Unbundle(w450) -> ()  [unwired: 3 out]
        n212 = Index Array(array=w445, index (row)=0, index (col)=0) -> (element=w443:sgl)
        n213 = local read "高负"() -> (w444:sgl)
        n214 = Multiply(x=w443, y=-1.004) -> (x*y=w441:dbl)
        n215 = Bundle(w441, "高负"=w444) -> (w440:cluster{dbl, "高负":sgl})  [unwired: 1 in]
      }
      frame 3 {
        w466 = FALSE
        n216 = Build Array(w466, w466, w466, TRUE, w466, w466, w466, w466) -> (w482:bool[])
        n217 = Boolean Array To Number(Boolean array=w482) -> (number=w487:u32)
        n218 = To Unsigned Byte Integer(number=w487) -> (unsigned 8bit integer=w486:u8)
        n219 = call "StartRead.vi"("错误输入（无错误）"=w480, "DevIndex"=w481) -> ("错误输出"=w483:errorcluster, "DevIndex Output"=w484:i32)  [unwired: 8 in]
        n220 = call "SetDioOut.vi"("错误输入（无错误）"=w483, "DioOut"=w486, "DioChanSel"=u8 255, "DevIndex"=w484) -> ("错误输出"=w476:errorcluster, "DevIndex Output"=w477:i32)  [unwired: 6 in]
        n221 = call "GetAiChans.vi"("错误输入（无错误）"=w476, "Num"=u32 1, "ChanSel"=u16 4, "DevIndex"=w477) -> ("错误输出"=w474:errorcluster, "Ai"=w471:sgl[][], "DevIndex Output"=w475:i32)  [unwired: 4 in, 1 out]
        n222 = Unbundle(w476) -> ()  [unwired: 3 out]
        n223 = Index Array(array=w471, index (row)=0, index (col)=0) -> (element=w469:sgl)
        n224 = local read "低正"() -> (w470:sgl)
        n225 = Divide(x=w469, y=2.564) -> (x/y=w467:dbl)
        n226 = Bundle(w467, "低正"=w470) -> (w464:cluster{dbl, "低正":sgl})  [unwired: 1 in]
      }
      frame 4 {
        w489 = FALSE
        n227 = call "StartRead.vi"("错误输入（无错误）"=w504, "DevIndex"=w505) -> ("错误输出"=w507:errorcluster, "DevIndex Output"=w508:i32)  [unwired: 8 in]
        n228 = local read "低负"() -> (w493:sgl)
        n229 = Build Array(w489, w489, w489, w489, w489, TRUE, w489, w489) -> (w506:bool[])
        n230 = Boolean Array To Number(Boolean array=w506) -> (number=w511:u32)
        n231 = To Unsigned Byte Integer(number=w511) -> (unsigned 8bit integer=w510:u8)
        n232 = call "SetDioOut.vi"("错误输入（无错误）"=w507, "DioOut"=w510, "DioChanSel"=u8 255, "DevIndex"=w508) -> ("错误输出"=w499:errorcluster, "DevIndex Output"=w500:i32)  [unwired: 6 in]
        n233 = Unbundle(w499) -> ()  [unwired: 3 out]
        n234 = call "GetAiChans.vi"("错误输入（无错误）"=w499, "Num"=u32 1, "ChanSel"=u16 8, "DevIndex"=w500) -> ("错误输出"=w498:errorcluster, "Ai"=w494:sgl[][], "DevIndex Output"=w497:i32)  [unwired: 4 in, 1 out]
        n235 = Index Array(array=w494, index (row)=0, index (col)=0) -> (element=w492:sgl)
        n236 = Divide(x=w492, y=-2.294) -> (x/y=w490:dbl)
        n237 = Bundle(w490, "低负"=w493) -> (w488:cluster{dbl, "低负":sgl})  [unwired: 1 in]
      }
      frame 5 {
        w513 = 0.0
        (unwired) TRUE
        w516 = FALSE
        n238 = call "StartRead.vi"("错误输入（无错误）"=w517, "DevIndex"=w518) -> ("错误输出"=w520:errorcluster, "DevIndex Output"=w521:i32)  [unwired: 8 in]
        n239 = Build Array(w516, w516, w516, w516, w516, w516, w516, w516) -> (w519:bool[])
        n240 = Boolean Array To Number(Boolean array=w519) -> (number=w524:u32)
        n241 = To Unsigned Byte Integer(number=w524) -> (unsigned 8bit integer=w523:u8)
        n242 = call "SetDioOut.vi"("错误输入（无错误）"=w520, "DioOut"=w523, "DioChanSel"=u8 255, "DevIndex"=w521) -> ("错误输出"=w514:errorcluster, "DevIndex Output"=w515:i32)  [unwired: 6 in]
        n243 = Unbundle(w514) -> ()  [unwired: 3 out]
        n244 = Bundle(w513, w513) -> (w512:cluster{dbl, dbl})  [unwired: 1 in]
      }
    }
    "输出气压波形图表" <- w267
    n245 = Unbundle(w267) -> (→"测量值":dbl, "高正"=→"给定值":dbl)
    n246 = case shown="真" "自动破膜" {
      frame False {
      }
      frame True {
        n247 = local read "阻值数组"() -> (w315:dbl[])
        n248 = Index Array(array=w315, index=0 ("索引")) -> (element=w311:dbl)
        n249 = Less?(x=500.0 ("y"), y=w311) -> (x < y?=w313:bool)
        n250 = case shown="真" w313 {
          frame False {
            n251 = local write "自动破膜"(FALSE) -> ()
          }
          frame True {
            n252 = case shown="\"200ms\", 默认" "枚举" {
              tunnel: [200.0 1000.0 500.0] -> w317
              frame "200ms", Default {
              }
              frame "1000ms" {
              }
              frame "500ms" {
              }
            }
            n253 = Tick Count (ms)() -> (millisecond timer value=w319:u32)
            n254 = local read "起始破膜时间"() -> (w322:u32)
            n255 = Subtract(x=w319, y=w322) -> (x-y=w320:u32)
            n256 = Greater?(x=w317, y=w320) -> (0:w321:bool)
            n257 = case shown="假" w321 {
              frame False {
                n258 = flat-sequence {
                  frame #0 {
                    w328 = FALSE
                    n259 = local write "高负开关"(w328) -> ()
                    n260 = local write "低正开关"(w328) -> ()
                    n261 = local write "高正开关"(w328) -> ()
                    n262 = local write "低负开关"(w328) -> ()
                    n263 = local write "大气压"(TRUE) -> ()
                    n264 = local write "case"(5.0) -> ()
                  }
                  frame #1 {
                    n265 = local write "自动破膜"(FALSE ("自动破膜")) -> ()
                    n266 = One Button Dialog(message="恭喜你，成功破膜" ("消息")) -> ()  [unwired: 1 in, 1 out]
                  }
                }
              }
              frame True {
                n267 = flat-sequence {
                  frame #0 {
                    w333 = FALSE
                    n268 = local write "高负开关"(TRUE) -> ()
                    n269 = local write "低正开关"(w333) -> ()
                    n270 = local write "高正开关"(w333) -> ()
                    n271 = local write "低负开关"(w333) -> ()
                    n272 = local write "大气压"(w333) -> ()
                    n273 = local write "case"(2.0) -> ()
                  }
                  frame #1 {
                    n274 = local write "高负"(-5.0) -> ()
                  }
                }
              }
            }
          }
        }
      }
    }
  }
  n275 = while {
    tunnel: w129 -> [w534]
    tunnel: [w533] -> w61
    tunnel: w27 -> [w532]
    tunnel: w26 -> [w531]
    stop <- w529 stop-if-true
    # "电流信号循环"
    n276 = Dequeue Element(queue=w532, timeout in ms (-1)=1 ("超时毫秒(-1)"), error in (no error)=w531) -> (error out=w527:errorcluster)  [unwired: 3 out]
    n277 = Unbundle By Name(w527) -> ("status"=w529:bool)
    n278 = flat-sequence {
      tunnel: w534 -> [w555]
      tunnel: [w555] -> w526
      tunnel: [w543] -> w525
      tunnel: [w563] -> w536
      tunnel: [w578] -> w535
      tunnel: w526 -> [w564]
      tunnel: w525 -> [w578]
      tunnel: [w599] -> w540
      tunnel: [w584] -> w539
      tunnel: w536 -> [w579]
      tunnel: w535 -> [w595]
      tunnel: w540 -> [w674]
      tunnel: w539 -> [w675]
      tunnel: w534 -> [w676]
      tunnel: [w673] -> w538
      tunnel: [w665] -> w537
      tunnel: [w718] -> w533
      tunnel: w538 -> [w718]
      tunnel: w537 -> [w716]
      frame #0 {
        n279 = case shown="假" "控制箱刺激ON\n/放大器刺激" {
          tunnel: [0.0 ("data") 5.0 ("data")] -> w552
          frame False {
          }
          frame True {
          }
        }
        n280 = call-poly <vilib>:"DAQmx Create Virtual Channel.vi"("physical channels"=tag "Dev2/ao1") -> ("task out"=w548:refnum<k21>, "error out"=w549:errorcluster)  [unwired: 13 in]
        n281 = call <vilib>:"DAQmx Start Task.vi"("task/channels in"=w548, "error in"=w549) -> ("task out"=w547:refnum<k21>, "error out"=w546:errorcluster)  [unwired: 12 in]
        n282 = call-poly <vilib>:"DAQmx Write.vi"("task/channels in"=w547, "data"=w552, "error in"=w546) -> ("task out"=w545:refnum<k21>, "error out"=w544:errorcluster)  [unwired: 10 in, 1 out]
        n283 = call <vilib>:"DAQmx Stop Task.vi"("task/channels in"=w545, "error in"=w544) -> ("task out"=w551:refnum<k21>, "error out"=w550:errorcluster)  [unwired: 12 in]
        n284 = call <vilib>:"DAQmx Clear Task.vi"("task in"=w551, "error in"=w550) -> ("error out"=w543:errorcluster)  [unwired: 13 in]
      }
      frame #1 {
        n285 = Unbundle By Name(w564) -> ("amplitude"=w570:dbl, "frequency"=w569:dbl, "Fs"=w571:dbl, "Averaging"=w572:i32)
        n286 = Multiply(x=w571, y=w572) -> (x*y=w567:dbl)
        n287 = Multiply(x="钳制电位", y="Holding Voltage") -> (x*y=w560:dbl)
        n288 = Divide(x=w567, y=w569) -> (x/y=w568:dbl)
        n289 = Divide(x=w570, y=2.0) -> (x/y=w574:dbl)
        n290 = Add(x=w560, y=0.5) -> (x+y=w558:dbl)
        "x*y" <- w558
        n291 = Divide(x=w558, y=1000.0) -> (x/y=w575:dbl)
        n292 = Add(x=w575, y=w574) -> (x+y=w565:dbl)
        n293 = Bundle("Fs"=w571, w568) -> (w573:cluster{"Fs":dbl, dbl})  [unwired: 1 in]
        n294 = call <vilib>:"Basic Function Generator.vi"("offset"=w565, "sampling info"=w573, "signal type"=T10."Square Wave", "amplitude"=w574, "frequency"=w569) -> ("signal out"=w563:waveform(dbl))  [unwired: 4 in, 2 out]
      }
      frame #2 {
        w628 = 10178 items=["有限采样"=10178, "连续采样"=10123, "硬件定时单点"=12522] ("sample mode")
        w629 = tag "OnboardClock" ("source")
        w621 = 10178 items=["有限采样"=10178, "连续采样"=10123, "硬件定时单点"=12522] ("sample mode")
        # "必须要有触发"
        # "This version of StimRecord is for the NI DAQ used in conjunction with the MultiClamp 700b"
        # "multiclamp放大器自己参数"
        # "in V"
        # "in nA"
        n295 = case shown="0, 默认" "电压钳/电流钳" {
          tunnel: [50.0 ("y") 2500000000.0 ("y")] -> w596
          tunnel: [2000.0 ("y") 0.1 ("y")] -> w597
          frame 0, Default {
          }
          frame 1 {
          }
        }
        n296 = Multiply(x=w579, y=w596) -> (x*y=w614:waveform(dbl))
        n297 = call-poly <vilib>:"Waveform Duration.vi"("waveform in"=w579) -> ("duration"=w616:dbl)  [unwired: 8 in, 2 out]
        n298 = Unbundle By Name(w614) -> ("Y"=w583:dbl[], "dt"=w613:dbl)
        n299 = for {
          tunnel: [w643] -> w582 mode=indexing
          tunnel: w583 -> [w637] mode=indexing
          w638 = 10.0 ("t")
          w641 = -10.0 ("t")
          n300 = Greater?(x=w641, y=w637) -> (0:w642:bool)
          n301 = Select(t=w641, s=w642, f=w637) -> (s? t:f=w639:dbl)
          n302 = Less?(x=w638, y=w639) -> (x < y?=w640:bool)
          n303 = Select(t=w638, s=w640, f=w639) -> (s? t:f=w643:dbl)
        }
        n304 = Multiply(x=w616, y=2.0) -> (x*y=w617:dbl)
        n305 = Add(x=w617, y=5.0) -> (x+y=w586:dbl)
        n306 = call-poly <vilib>:"DAQmx Create Virtual Channel.vi"("physical channels"=tag "Dev2/ai0", "error in"=w595) -> ("task out"=w620:refnum<k21>, "error out"=w619:errorcluster)  [unwired: 12 in]
        n307 = call-poly <vilib>:"DAQmx Create Virtual Channel.vi"("physical channels"=tag "Dev2/ao0", "error in"=w595) -> ("task out"=w609:refnum<k21>, "error out"=w608:errorcluster)  [unwired: 12 in]
        n308 = Reciprocal(x=w613) -> (1/x=w622:dbl)
        n309 = Array Size(array=w583) -> (size(s)=w636:i32)
        n310 = call-poly <vilib>:"DAQmx Timing.vi"("task/channels in"=w609, "sample mode"=w628, "samples per channel"=w636, "rate"=w622, "source"=w629, "error in"=w608) -> ("task out"=w594:refnum<k21>, "error out"=w592:errorcluster)  [unwired: 8 in]
        n311 = Bundle By Name(cluster=w614, "Y"=w582) -> (w615:waveform(dbl))
        n312 = call-poly <vilib>:"DAQmx Timing.vi"("task/channels in"=w620, "sample mode"=w621, "samples per channel"=w636, "rate"=w622, "source"=w629, "error in"=w619) -> ("task out"=w624:refnum<k21>, "error out"=w625:errorcluster)  [unwired: 8 in]
        n313 = call-poly <vilib>:"DAQmx Trigger.vi"("task/channels in"=w594, "source"=tag "/Dev2/ai/StartTrigger", "error in"=w592) -> ("task out"=w593:refnum<k21>, "error out"=w591:errorcluster)  [unwired: 11 in]
        n314 = call-poly <vilib>:"DAQmx Write.vi"("task/channels in"=w593, "auto start"=FALSE, "data"=w615, "timeout"=w586, "error in"=w591) -> ("task out"=w612:refnum<k21>, "error out"=w633:errorcluster)  [unwired: 8 in, 1 out]
        n315 = property class="DAQmx定时" props=["SampClk.Rate"](reference=w624, error in=w625) -> (reference out=w626:refnum<k21>)  [unwired: 2 out]
        n316 = call <vilib>:"DAQmx Start Task.vi"("task/channels in"=w612, "error in"=w633) -> ("task out"=w630:refnum<k21>, "error out"=w632:errorcluster)  [unwired: 12 in]
        n317 = call <vilib>:"DAQmx Start Task.vi"("task/channels in"=w626, "error in"=w632) -> ("task out"=w604:refnum<k21>, "error out"=w605:errorcluster)  [unwired: 12 in]
        n318 = call-poly <vilib>:"DAQmx Read.vi"("task/channels in"=w604, "number of samples per channel"=w636, "timeout"=w586, "error in"=w605) -> ("task out"=w590:refnum<k21>, "data"=w618:waveform(dbl), "error out"=w588:errorcluster)  [unwired: 9 in]
        n319 = call <vilib>:"DAQmx Is Task Done.vi"("task/channels in"=w630, "error in"=w632) -> ("task out"=w631:refnum<k21>, "error out"=w634:errorcluster)  [unwired: 11 in, 1 out]
        n320 = call <vilib>:"DAQmx Wait Until Done.vi"("task/channels in"=w631, "timeout (sec)"=w586, "error in"=w634) -> ("task out"=w610:refnum<k21>, "error out"=w611:errorcluster)  [unwired: 11 in]
        n321 = call <vilib>:"DAQmx Wait Until Done.vi"("task/channels in"=w590, "timeout (sec)"=w586, "error in"=w588) -> ("task out"=w589:refnum<k21>, "error out"=w587:errorcluster)  [unwired: 11 in]
        n322 = call <vilib>:"DAQmx Stop Task.vi"("task/channels in"=w610, "error in"=w611) -> ("task out"=w607:refnum<k21>, "error out"=w606:errorcluster)  [unwired: 12 in]
        n323 = Multiply(x=w618, y=w597) -> (x*y=w584:waveform(dbl))
        "电流信号波形图" <- w584
        n324 = call <vilib>:"DAQmx Stop Task.vi"("task/channels in"=w589, "error in"=w587) -> ("task out"=w602:refnum<k21>, "error out"=w603:errorcluster)  [unwired: 12 in]
        n325 = call <vilib>:"DAQmx Clear Task.vi"("task in"=w607, "error in"=w606) -> ("error out"=w635:errorcluster)  [unwired: 13 in]
        n326 = call <vilib>:"DAQmx Clear Task.vi"("task in"=w602, "error in"=w603) -> ("error out"=w601:errorcluster)  [unwired: 13 in]
        n327 = Merge Errors(w635, w601) -> (w599:errorcluster)
        n328 = Build Array(w614, w584) -> ()  [unwired: 1 out]
      }
      frame #3 {
        # "数据读取错误"
        # "阻值读取异常处理"
        # "单位换算不明白"
        # "阻值处理"
        # "Convert Volts/pA into MOhms"
        n329 = call "Filter"("error in (no error)"=w674, "Signal"=w675) -> ("error out"=w677:errorcluster, "Filtered Signal"=w669:dynamicdata)  [unwired: 8 in]
        n330 = call "单频测量"("Signals"=w669) -> ("Frequency"=w668:dynamicdata)  [unwired: 9 in, 1 out]
        n331 = Unbundle By Name(w676) -> ("Fs"=w690:dbl, "frequency"=w689:dbl, "Proportion"=w682:dbl)
        n332 = Unbundle By Name(w676) -> ("Averaging"=w688:i32)
        n333 = call "Convert from Dynamic Data"("Dynamic Data Type"=w669) -> ("Array"=w680:dbl[])  [unwired: 3 in]
        n334 = call "从动态数据转换"("Dynamic Data Type"=w668) -> ("Array"=w667:dbl[])  [unwired: 3 in]
        n335 = call-poly <vilib>:"Mean.vi"("X"=w667) -> ("mean"=w664:dbl)  [unwired: 1 out]
        n336 = Divide(x=w690, y=w689) -> (x/y=w693:dbl)
        n337 = Reshape Array(w680, w688, w693) -> (w692:dbl[][])
        n338 = call-poly <vilib>:"Mean.vi"("X"=w680) -> ("mean"=w681:dbl)  [unwired: 1 out]
        n339 = for {
          N: w688 -> [_]
          tunnel: w692 -> [w704] mode=indexing
          tunnel: w677 -> [w711]
          shift-right: [w712] -> w691
          shift-left: dbl[] [] -> [w713]
          tunnel: [w699] -> w687
          tunnel: [w711] -> w673
          tunnel: w682 -> [w703]
          # "不是整个电流的均值"
          # "波形后半段"
          # "波形前半段"
          n340 = Array Size(array=w704) -> (size(s)=w701:i32)
          n341 = Subtract(x=1.0, y=w703) -> (x-y=w706:dbl)
          n342 = Divide(x=w701, y=2) -> (x/y=w708:dbl)
          n343 = Multiply(x=w708, y=w706) -> (x*y=w705:dbl)
          n344 = Split 1D Array(array=w704, index=w708) -> (first subarray=w700:dbl[], second subarray=w709:dbl[])
          n345 = Split 1D Array(array=w700, index=w705) -> (second subarray=w696:dbl[])  [unwired: 1 out]
          n346 = Split 1D Array(array=w709, index=w705) -> (second subarray=w697:dbl[])  [unwired: 1 out]
          n347 = call-poly <vilib>:"Mean.vi"("X"=w696) -> ("mean"=w698:dbl)  [unwired: 1 out]
          n348 = call-poly <vilib>:"Mean.vi"("X"=w697) -> ("mean"=w699:dbl)  [unwired: 1 out]
          n349 = Subtract(x=w698, y=w699) -> (x-y=w702:dbl)
          n350 = Build Array (concatenate)(w713, w702) -> (w712:dbl[])
        }
        "Negative Peak" <- w687
        n351 = Subtract(x=w664, y=sgl 20.0) -> (x-y=w662:dbl)
        n352 = Array Max & Min(array=w680) -> (min value=w679:dbl)  [unwired: 3 out]
        n353 = Absolute Value(x=w662) -> (abs(x)=w661:dbl)
        n354 = Greater?(x=w661, y=0.05) -> (0:w655:bool)
        "！" <- w655
        n355 = Subtract(x=w681, y=w679) -> (x-y=w678:dbl)
        n356 = Unbundle By Name(w676) -> ("amplitude"=w685:dbl)
        n357 = Multiply(x=w685, y=1000000.0) -> (x*y=w672:dbl)
        n358 = Divide(x=w672, y=w678) -> (x/y=→"电阻值":dbl)
        n359 = call-poly <vilib>:"Mean.vi"("X"=w691) -> ("mean"=w686:dbl)  [unwired: 1 out]
        n360 = local read "Resistance(MΩ)"() -> (w658:dbl)
        n361 = Divide(x=w672, y=w686) -> (x/y=w671:dbl)
        n362 = Multiply(x=w671, y=2.0) -> (x*y=w670:dbl)
        n363 = local read "阻值数组"() -> (w666:dbl[])
        n364 = Less?(x=w658, y=100.0) -> (x < y?=w656:bool)
        n365 = And(x=w656, y=w655) -> (x .and. y?=w654:bool)
        n366 = case shown="假" w654 {
          tunnel: w658 -> [_ w695]
          tunnel: w670 -> [w694 _]
          tunnel: [w694 w695] -> w653
          frame False {
          }
          frame True {
          }
        }
        n367 = In Range and Coerce(upper limit=10000.0 ("上限"), x=w653, lower limit=0.0 ("下限")) -> (coerced(x)=w648:dbl)  [unwired: 1 out]
        "阻值波形图表" <- w648
        "Resistance(MΩ)" <- w648
        n368 = Insert Into Array(array=w666, index=0 ("索引"), new element=w648) -> (w665:dbl[])
        n369 = local write "阻值数组"(w665) -> ()
      }
      frame #4 {
        n370 = Array Size(array=w716) -> (size(s)=w715:i32)
        n371 = Greater?(x=w715, y=10) -> (0:w714:bool)
        n372 = case shown="真" w714 {
          tunnel: w716 -> [_ w722]
          frame False {
          }
          frame True {
            n373 = Delete From Array(array=w722, length=1 ("长度"), index=9 ("索引")) -> (array with subset deleted=w719:dbl[])  [unwired: 1 out]
            n374 = local write "阻值数组"(w719) -> ()
          }
        }
      }
    }
    n375 = case shown="真" "入液阻值校准" {
      frame False {
      }
      frame True {
        n376 = flat-sequence {
          frame #0 {
            n377 = local read "Resistance(MΩ)"() -> (→"校准的入液阻值":dbl)
          }
          frame #1 {
            n378 = local write "入液阻值校准"(FALSE) -> ()
          }
        }
      }
    }
  }
  n379 = VISA Close(VISA resource name=w29, error in (no error)=w28) -> ()  [unwired: 1 out]
  n380 = call "IMAQ Create"("Image Name"="针尖图像处理") -> ("New Image"=w64:T4)  [unwired: 4 in, 1 out]
  n381 = call "IMAQ Create"("Image Name"="二值化") -> ("New Image"=w63:T4)  [unwired: 4 in, 1 out]
  n382 = call "IMAQ Create"("Image Name"="镜像") -> ("New Image"=w6:T4)  [unwired: 4 in, 1 out]
  n383 = call "IMAQ Create"("Image Name"="", "Image Type"=w16) -> ("New Image"=w13:T4)  [unwired: 3 in, 1 out]
  n384 = call "IMAQ Create"("Image Name"="", "Image Type"=w14) -> ("New Image"=w12:T4)  [unwired: 3 in, 1 out]
  n385 = call "IMAQ Create"("Image Name"="旋转") -> ("New Image"=w8:T4)  [unwired: 4 in, 1 out]
  n386 = call "IMAQ Create"("Image Name"="unet裁剪") -> ("New Image"=w34:T4)  [unwired: 4 in, 1 out]
  n387 = call "IMAQ Create"("Image Name"="mask图像") -> ("New Image"=w32:T4)  [unwired: 4 in, 1 out]
  n388 = while {
    tunnel: w139 -> [w765]
    tunnel: w137 -> [w764]
    tunnel: [w737] -> w132
    shift-right: [w762] -> _
    shift-left: _ -> [w761]
    tunnel: w130 -> [w759]
    tunnel: [w747] -> w128
    tunnel: [w758] -> w127
    tunnel: w126 -> [w757]
    tunnel: [w756] -> w125
    tunnel: w124 -> [w755]
    tunnel: w27 -> [w754]
    tunnel: [w751] -> w122
    shift-right: [w750] -> w121
    shift-left: w26 -> [w749]
    tunnel: w67 -> [w748]
    tunnel: w64 -> [w746]
    tunnel: w63 -> [w745]
    tunnel: w34 -> [w736]
    tunnel: w32 -> [_]
    tunnel: w8 -> [w733]
    tunnel: w6 -> [w732]
    tunnel: w2 -> [w731]
    stop <- "停止" stop-if-true
    # "图像检测"
    # "图像处理循环"
    n389 = disable-structure shown="禁用" {
      frame Disabled {
        (unwired) 2 ("长度")
        # "目标坐标"
        n390 = property on="Image" class="ImageControl"() -> ("ROI"=w766:T11)  [unwired: 2 in, 2 out]
        n391 = Unbundle(w766) -> ("Global Rectangle"=w768:i32[])  [unwired: 1 out]
        n392 = Array Subset(array=w768, index=0 ("索引")) -> (→"目标坐标":i32[])  [unwired: 1 in]
      }
      frame Enabled {
      }
    }
    n393 = Tick Count (ms)() -> (millisecond timer value=w762:u32)
    n394 = call <vilib>:"IMAQdx Grab2.vi"("error in"=w757, "Image In"=w764, "Session In"=w765) -> ("error out"=w756:errorcluster, "Image Out"=w760:T4, "Session Out"=w737:T6)  [unwired: 5 in, 1 out]
    n395 = Subtract(x=w762, y=w761) -> (x-y=→"循环时间":u32)
    n396 = call "IMAQ ExtractSingleColorPlane"("error in (no error)"=w755, "Image Dst"=w759, "Image Src"=w760) -> ("error out"=w758:errorcluster, "Image Dst Out"=w747:T4)  [unwired: 7 in]
    n397 = Enqueue Element(queue=w754, element="停止", timeout in ms (-1)=1 ("超时毫秒(-1)"), error in (no error)=w749) -> (queue out=w751:refnum<queue>, error out=w750:errorcluster)  [unwired: 1 out]
    n398 = local read "针尖自动移动 2"() -> (w727:bool)
    n399 = local read "针尖自动移动"() -> (w728:bool)
    n400 = local read "针尖细对焦"() -> (w729:bool)
    n401 = local read "升Z轴找针"() -> (w726:bool)
    n402 = Or(x=w729, y=w728) -> (x .or. y?=w725:bool)
    n403 = Or(x=w725, y="针尖模板匹配") -> (x .or. y?=w723:bool)
    n404 = Compound Arithmetic op=OR("针尖模板匹配", w729, w726, w728, w727) -> (w730:bool)
    n405 = case shown="真" w730 {
      tunnel: w748 -> [_ w963]
      tunnel: w747 -> [w957 w966]
      tunnel: [FALSE w1001] -> w741
      tunnel: [w956 w969] -> _
      tunnel: [w957 w965] -> w740
      tunnel: w731 -> [_ w961]
      tunnel: w723 -> [_ w960]
      frame False {
        w958 = 0.0 ("x")
        n406 = Bundle("x"=w958, "x"=w958) -> (w956:cluster{"x":dbl, "x":dbl})  [unwired: 1 in]
      }
      frame True {
        w968 = u32 1 items=["Frame", "Fill", "Highlight"] ("Drawing Mode (Frame)")
        w971 = 10.0 ("y")
        w995 = u16 0 items=["All", "Shift Information", "Rotation Information"] ("Learn Mode")
        # "目标和针尖坐标获取"
        # "模板针尖偏移量"
        # "是否匹配到"
        # "模板匹配针尖"
        n407 = case shown="真" w960 {
          tunnel: [w1002 w1003] -> w962
          tunnel: w963 -> [_ w1003]
          tunnel: w961 -> [w1002 _]
          frame False {
          }
          frame True {
          }
        }
        n408 = call "IMAQ Setup Match Pattern 2"("Minimum Contrast"="Minimum Contrast", "Match Mode"="Match Mode") -> ("Match Pattern Setup Data"=w999:string)  [unwired: 8 in, 1 out]
        n409 = call "IMAQ Setup Learn Pattern 2"("Learn Mode"=w995) -> ("Learn Pattern Setup Data"=w994:string)  [unwired: 9 in, 1 out]
        n410 = call "IMAQ Learn Pattern 2"("Learn Pattern Setup Data"=w994, "Image"=w962) -> ("Template Image Out"=w991:T4)  [unwired: 8 in, 1 out]
        n411 = call "IMAQ Match Pattern 2"("Minimum Match Score"="Minimum Match Score", "Number of Matches Requested"="Number of Matches Requested", "Match Pattern Setup Data"=w999, "Template Image"=w991, "Image"=w966) -> ("Number of Matches"=w992:i32, "Matches"=w988:T1)  [unwired: 4 in, 1 out]
        "Number of Matches" <- w992
        "Matches 2" <- w988
        n412 = Equal?(x=w992, y=0) -> ()  [unwired: 1 out]
        n413 = Index Array(array=w988, index=0 ("索引")) -> (element=w986:T12)
        n414 = Index Array(array=w988, index=0 ("索引")) -> (element=w970:T12)
        n415 = Unbundle(w986) -> ("Score"=w985:sgl)  [unwired: 4 out]
        n416 = Less?(x=w985, y=sgl 780.0) -> (x < y?=w1001:bool)
        n417 = Unbundle(w970) -> ("Position"=w969:cluster{"x":sgl, "y":sgl})  [unwired: 4 out]
        n418 = Cluster To Array(cluster=w969) -> (array=→"针尖坐标":sgl[])
        n419 = Unbundle(w969) -> ("x"=w980:sgl, "y"=w983:sgl)
        n420 = Add(x=w980, y=sgl 0.0) -> (x+y=w982:sgl)
        n421 = Subtract(x=w983, y=w971) -> (x-y=w974:dbl)
        n422 = Add(x=w983, y=w971) -> (x+y=w973:dbl)
        n423 = Subtract(x=w982, y=w971) -> (x-y=w972:dbl)
        n424 = Add(x=w982, y=w971) -> (x+y=w975:dbl)
        n425 = To Long Integer(number=w974) -> (32bit integer=w977:i32)
        n426 = To Long Integer(number=w973) -> (32bit integer=w978:i32)
        n427 = To Long Integer(number=w972) -> (32bit integer=w976:i32)
        n428 = To Long Integer(number=w975) -> (32bit integer=w979:i32)
        n429 = Bundle(w976, w977, w979, w978) -> (w967:cluster{i32, i32, i32, i32})  [unwired: 1 in]
        n430 = call "IMAQ Overlay Oval"("Color"=u32 6618880, "Drawing Mode (Frame)"=w968, "Bounding Rectangle"=w967, "Image"=w966) -> ("Image Out"=w965:T4)  [unwired: 6 in, 1 out]
      }
    }
    "Image" <- w740
    "是否匹配到？" <- w741
    n431 = local read "针尖细对焦"() -> (w742:bool)
    n432 = local read "针尖粗对焦"() -> (w743:bool)
    n433 = local read "自动扫描"() -> (w739:bool)
    n434 = Or(x=w743, y=w742) -> (x .or. y?=w738:bool)
    n435 = Or(x=w739, y=w738) -> ()  [unwired: 1 out]
    n436 = case shown="真" TRUE {
      tunnel: [0.0 ("Right") w913] -> w744
      tunnel: w740 -> [_ w946]
      tunnel: w746 -> [_ w945]
      tunnel: w745 -> [_ w944]
      tunnel: w733 -> [_ _]
      tunnel: w732 -> [_ w929]
      frame False {
      }
      frame True {
        w930 = u32 0 items=["Horizontal", "Vertical", "Central", "1st Diagonal", "2nd Diagonal"] ("Type of Symmetry")
        # "目标标定"
        n437 = call "IMAQ Threshold"("Range"="Range", "Image Dst"=w944, "Image Src"=w946) -> ("Image Dst Out"=w947:T4)  [unwired: 7 in, 1 out]
        n438 = call "IMAQ LowPass"("Image Src"=w947) -> ("Image Dst Out"=w948:T4)  [unwired: 6 in, 1 out]
        n439 = call "IMAQ Copy"("Image Dst"=w945, "Image Src"=w948) -> ("Image Dst Out"=w954:T4)  [unwired: 4 in, 1 out]
        n440 = call "IMAQ RemoveParticle"("Number of Erosion"="Number of Erosion", "Image Src"=w954) -> ("Image Dst Out"=w949:T4)  [unwired: 8 in, 1 out]
        n441 = call "IMAQ Morphology"("Operation"="Operation", "Image Src"=w949) -> ("Image Dst Out"=w951:T4)  [unwired: 8 in, 1 out]
        n442 = call "IMAQ Convex Hull"("Image Src"=w951) -> ("Image Dst Out"=w952:T4)  [unwired: 9 in, 1 out]
        n443 = call "IMAQ FillHole"("Image Src"=w952) -> ("Image Dst Out"=w950:T4)  [unwired: 5 in, 1 out]
        n444 = call "IMAQ Clear Overlay"("Image"=w950) -> ("Image Out"=w922:T4)  [unwired: 9 in, 1 out]
        n445 = call "IMAQ ImageToArray"("Image"=w922) -> ("Image Pixels (U8)"=w920:u8[][])  [unwired: 3 in, 4 out]
        n446 = Transpose Matrix(1:w920) -> (0:w931:dbl[][])
        n447 = call "IMAQ ArrayToImage"("Image Pixels (U8)"=w931, "Image"=w929) -> ("Image Out"=w919:T4)  [unwired: 8 in, 1 out]
        n448 = call "IMAQ Symmetry"("Type of Symmetry"=w930, "Image Src"=w919) -> ("Image Dst Out"=w917:T4)  [unwired: 3 in, 1 out]
        "二值化" <- w917
        n449 = call "IMAQ Particle Analysis"("Pixel Measurements"="Pixel Measurements", "Image"=w917) -> ("Particle Measurements (Pixels)"=w932:dbl[][])  [unwired: 4 in, 5 out]
        "Particle Measurements (Pixels)" <- w932
        n450 = call "IMAQ Particle Analysis"("Pixel Measurements"="Pixel Measurements 2", "Image"=w917) -> ("Particle Measurements (Pixels)"=w915:dbl[][])  [unwired: 4 in, 5 out]
        "Particle Measurements (Pixels) 2" <- w915
        n451 = Array Max & Min(array=w932) -> (min value=w924:dbl)  [unwired: 3 out]
        n452 = Subtract(x=3072.0, y=w924) -> (x-y=w913:dbl)
        "Right" <- w913
        n453 = Array Max & Min(array=w915) -> (max value=w928:dbl, min value=w927:dbl)  [unwired: 2 out]
        n454 = Add(x=w928, y=w927) -> (x+y=w926:dbl)
        n455 = Greater?(x=w913, y=500.0) -> (0:w937:bool)
        n456 = Divide(x=w926, y=2.0) -> (x/y=w914:dbl)
        "startY" <- w914
        n457 = Greater?(x=w914, y=200.0) -> (0:w943:bool)
        n458 = Less?(x=w914, y=1600.0) -> (x < y?=w942:bool)
        n459 = Less?(x=w913, y=2500.0) -> (x < y?=w938:bool)
        n460 = And(x=w943, y=w942) -> (x .and. y?=w935:bool)
        n461 = And(x=w937, y=w938) -> (x .and. y?=w934:bool)
        n462 = And(x=w935, y=w934) -> (x .and. y?=w933:bool)
        n463 = local write "手动暂停"(w933) -> ()
      }
    }
    "清晰度评价函数" <- w744
    n464 = case shown="真" "图像网络检测" {
      tunnel: w736 -> [_ w770]
      frame False {
      }
      frame True {
        n465 = stacked-sequence {
          tunnel: w770 -> [_ _ _ w806 _ _]
          frame #0 {
            n466 = local read "Image"() -> (w772:T4)
            n467 = call-poly "IMAQ Write File 2"("File Path"=path "D:/faster-rcnn.pytorch-pytorch-1.0/temp_img/img.png", "Image"=w772) -> ()  [unwired: 8 in, 2 out]
          }
          frame #1 {
            n468 = Wait (ms)(milliseconds to wait=u32 100 ("等待时间（毫秒）")) -> ()  [unwired: 1 out]
          }
          frame #2 {
            w781 = 100 ("y")
            n469 = Open/Create/Replace File(file path (use dialog)=path "D:/faster-rcnn.pytorch-pytorch-1.0/data.txt" ("文件路径（使用对话框）")) -> (refnum out=w785:refnum<file>)  [unwired: 5 in, 2 out]
            n470 = Set File Position(refnum=w785, from (0:start)=enum16{"start", "end", "current"}."start" ("自（0:起始）")) -> (refnum out=w796:refnum<file>, error out=w798:errorcluster)  [unwired: 2 in]
            n471 = Read from Text File(file (use dialog)=w796, count=1 ("计数"), error in=w798) -> (refnum out=w784:refnum<file>, text=w787:string[])  [unwired: 1 in, 2 out]
            n472 = Close File(refnum=w784) -> ()  [unwired: 1 in, 2 out]
            n473 = Index Array(array=w787, index=0 ("索引")) -> (element=w778:string)
            n474 = Match Pattern(string=w778, regular expression="," ("正则表达式")) -> (before substring=w777:string, after substring=w776:string)  [unwired: 1 in, 2 out]
            n475 = Decimal String To Number(string=w777) -> (offset past number=w780:i32, number=→"X 2":i32)  [unwired: 2 in]
            n476 = Decimal String To Number(string=w776) -> (number=w789:i32)  [unwired: 2 in, 1 out]
            "Y 2" <- w789
            n477 = Subtract(x=w780, y=w781) -> (x-y=w782:i32)
            n478 = Subtract(x=w789, y=w781) -> (x-y=w793:i32)
            n479 = Add(x=w780, y=w781) -> (x+y=w794:i32)
            n480 = Add(x=w789, y=w781) -> (x+y=w792:i32)
            n481 = To Long Integer(number=w782) -> (32bit integer=w783:i32)
            n482 = To Long Integer(number=w793) -> (32bit integer=w775:i32)
            n483 = To Long Integer(number=w794) -> (32bit integer=w774:i32)
            n484 = To Long Integer(number=w792) -> (32bit integer=w791:i32)
            n485 = Build Array(w783, w775, w774, w791) -> (→"裁剪数组":i32[])
          }
          frame #3 {
            w802 = -1 ("y")
            n486 = local read "Y 2"() -> (w803:i32)
            n487 = local read "X 2"() -> (w800:i32)
            n488 = Equal?(x=w800, y=w802) -> (x = y?=w804:bool)
            n489 = Equal?(x=w803, y=w802) -> (x = y?=w805:bool)
            n490 = Or(x=w804, y=w805) -> (x .or. y?=w801:bool)
            n491 = case shown="真" w801 {
              tunnel: w806 -> [w824 _]
              frame False {
                (unwired) "hello" ("数据输入")
                (unwired) "10.134.224.218" ("名称")
                # "tcp通信"
                # "tcp通信"
                n492 = local read "裁剪数组"() -> (w823:i32[])
                n493 = local read "Image"() -> (w825:T4)
                n494 = call "IMAQ Extract 2"("Optional Rectangle"=w823, "Image Dst"=w824, "Image Src"=w825) -> ("Image Dst Out"=w809:T4)  [unwired: 7 in, 1 out]
                n495 = call "IMAQ Resample"("X Resolution"=128, "Y Resolution"=128, "Image Src"=w809) -> ("Image Dst Out"=w808:T4)  [unwired: 7 in, 1 out]
                n496 = call "IMAQ ImageToArray"("Image"=w808) -> ("Image Pixels (U8)"=w819:u8[][])  [unwired: 3 in, 4 out]
                n497 = for {
                  tunnel: w819 -> [w851] mode=indexing
                  tunnel: [w850] -> w821 mode=indexing
                  n498 = for {
                    tunnel: w851 -> [w852] mode=indexing
                    tunnel: [w853] -> w850 mode=indexing
                    n499 = Less?(x=w852, y=u8 10) -> (x < y?=w854:bool)
                    n500 = case shown="假" w854 {
                      tunnel: [w856 w868] -> w853
                      tunnel: w852 -> [w857 w869]
                      frame False {
                        n501 = Less?(x=w857, y=u8 100) -> (x < y?=w858:bool)
                        n502 = case shown="真" w858 {
                          tunnel: w857 -> [w861 w863]
                          tunnel: [w860 w862] -> w856
                          frame False {
                            n503 = Number To Decimal String(number=w861) -> (decimal integer string=w860:string)  [unwired: 1 in]
                          }
                          frame True {
                            n504 = Number To Decimal String(number=w863) -> (decimal integer string=w865:string)  [unwired: 1 in]
                            n505 = Concatenate Strings("0" ("字符串"), w865) -> (w862:string)
                          }
                        }
                      }
                      frame True {
                        n506 = Number To Decimal String(number=w869) -> (decimal integer string=w867:string)  [unwired: 1 in]
                        n507 = Concatenate Strings("00" ("字符串"), w867) -> (w868:string)
                      }
                    }
                  }
                }
                n508 = Concatenate Strings(w821) -> (w818:string)
                n509 = TCP Open Connection(address="10.134.24.208" ("名称"), remote port or service name=u16 8888 ("远程端口或服务名称")) -> (connection ID=w817:refnum<k5>, error out=w816:errorcluster)  [unwired: 3 in]
                n510 = TCP Write(connection ID=w817, data in=w818, error in (no error)=w816) -> (connection ID out=w814:refnum<k5>, bytes written=→"写入的字节":i32, error out=w815:errorcluster)  [unwired: 1 in]
                n511 = case shown="无错误" w815 {
                  selector: w815 -> [w844 _]
                  tunnel: [w834 errorcluster {"status"=FALSE, "code"=0, "source"=""} ("error IO")] -> w813
                  tunnel: [w836 w848] -> w812
                  tunnel: w814 -> [w833 w848]
                  frame No Error {
                    w830 = 1.5625
                    n512 = TCP Read(connection ID=w833, bytes to read=7 ("读取的字节"), error in (no error)=w844) -> (connection ID out=w836:refnum<k5>, data out=w837:string, error out=w835:errorcluster)  [unwired: 2 in]
                    "数据输出 3" <- w837
                    n513 = case shown="无错误" w835 {
                      selector: w835 -> [w846 _]
                      tunnel: [w846 errorcluster {"status"=FALSE, "code"=0, "source"=""} ("error IO")] -> w834
                      frame No Error {
                      }
                      frame Error {
                      }
                    }
                    n514 = String Subset(string=w837, offset (0)=4 ("偏移量(0)"), length (rest)=3 ("长度（剩余）")) -> (substring=w838:string)
                    n515 = String Subset(string=w837, offset (0)=1 ("偏移量(0)"), length (rest)=3 ("长度（剩余）")) -> (substring=w841:string)
                    n516 = Decimal String To Number(string=w838) -> (number=w827:i32)  [unwired: 2 in, 1 out]
                    n517 = Decimal String To Number(string=w841) -> (number=w826:i32)  [unwired: 2 in, 1 out]
                    n518 = Multiply(x=w827, y=w830) -> (x*y=w831:dbl)
                    n519 = Multiply(x=w826, y=w830) -> (x*y=w832:dbl)
                    n520 = Round To Nearest(number=w831) -> (nearest integer value=→"Y 3":dbl)
                    n521 = Round To Nearest(number=w832) -> (nearest integer value=→"X 3":dbl)
                  }
                  frame Error {
                  }
                }
                "error IO" <- w813
                n522 = TCP Close Connection(connection ID=w812, error in (no error)=w813) -> ()  [unwired: 1 in, 2 out]
              }
              frame True {
              }
            }
          }
          frame #4 {
            w872 = -1 ("y")
            n523 = local read "X 3"() -> (w885:i32)
            n524 = local read "Y 3"() -> (w883:i32)
            n525 = local read "X 2"() -> (w876:i32)
            n526 = local read "Y 2"() -> (w875:i32)
            n527 = Equal?(x=w876, y=w872) -> (x = y?=w874:bool)
            n528 = Equal?(x=w875, y=w872) -> (x = y?=w873:bool)
            n529 = Equal?(x=w885, y=0) -> (x = y?=w881:bool)
            n530 = Equal?(x=w883, y=0) -> (x = y?=w880:bool)
            n531 = local read "Image"() -> (w879:T4)
            n532 = Or(x=w874, y=w873) -> (x .or. y?=w871:bool)
            n533 = And(x=w881, y=w880) -> (x .and. y?=w877:bool)
            n534 = Or(x=w877, y=w871) -> (x .or. y?=w870:bool)
            n535 = call "IMAQ Clear Overlay"("Image"=w879) -> ("Image Out"=w878:T4)  [unwired: 9 in, 1 out]
            n536 = case shown="假" w870 {
              tunnel: w878 -> [w895 _]
              frame False {
                w890 = u32 1 items=["Frame", "Fill"] ("Drawing Mode (Frame)")
                w901 = 10 ("y")
                n537 = local read "X 2"() -> (w899:i32)
                n538 = local read "X 3"() -> (w898:i32)
                n539 = local read "Y 2"() -> (w897:i32)
                n540 = local read "Y 3"() -> (w896:i32)
                n541 = Add(x=w899, y=w898) -> (x+y=w889:i32)
                n542 = Add(x=w897, y=w896) -> (x+y=w888:i32)
                n543 = Build Array(w889, w888) -> (w887:i32[])
                n544 = Subtract(x=w889, y=100) -> (x-y=w894:i32)
                n545 = Subtract(x=w888, y=100) -> (x-y=w891:i32)
                n546 = Subtract(x=w894, y=w901) -> (x-y=w902:i32)
                n547 = Add(x=w894, y=w901) -> (x+y=w905:i32)
                n548 = Subtract(x=w891, y=w901) -> (x-y=w904:i32)
                n549 = Add(x=w891, y=w901) -> (x+y=w903:i32)
                n550 = local write "目标坐标"(w887) -> ()
                n551 = To Long Integer(number=w902) -> (32bit integer=w906:i32)
                n552 = To Long Integer(number=w905) -> (32bit integer=w909:i32)
                n553 = To Long Integer(number=w904) -> (32bit integer=w907:i32)
                n554 = To Long Integer(number=w903) -> (32bit integer=w908:i32)
                n555 = Bundle(w906, w907, w909, w908) -> (w900:cluster{i32, i32, i32, i32})  [unwired: 1 in]
                n556 = call "IMAQ Overlay Oval"("Color"=u32 16711680, "Drawing Mode (Frame)"=w890, "Bounding Rectangle"=w900, "Image"=w895) -> ()  [unwired: 6 in, 2 out]
                "图像检测到" <- TRUE
              }
              frame True {
              }
            }
          }
          frame #5 {
            n557 = local write "图像网络检测"(FALSE) -> ()
          }
        }
      }
    }
  }
  n558 = Get Date/Time String(date format (0)=enum16{"short", "long", "abbreviated"}."long" ("日期格式(0)"), want seconds? (F)=TRUE ("需要秒？(F)")) -> (date string=w58:string, time string=w43:string)  [unwired: 1 in]
  n559 = String Subset(string=w43, offset (0)=6 ("偏移量(0)")) -> (substring=w41:string)  [unwired: 1 in]
  n560 = String Subset(string=w43, offset (0)=3 ("偏移量(0)"), length (rest)=2 ("长度（剩余）")) -> (substring=w53:string)
  n561 = String Subset(string=w43, length (rest)=2 ("长度（剩余）")) -> (substring=w55:string)  [unwired: 1 in]
  n562 = Concatenate Strings(w55, "时" ("字符串"), w53, "分" ("字符串"), w41, "秒" ("字符串")) -> (w54:string)
  n563 = Concatenate Strings(w58, w54) -> (w37:string)
  n564 = Build Path(base path=path "D:/韩宇/实验/数据" ("文件路径（使用对话框）"), name or relative path=w37) -> (appended path=w51:path)
  n565 = Create Folder(path (use dialog)=w51) -> (created path=w46:path)  [unwired: 2 in, 2 out]
  n566 = Build Path(base path=w46, name or relative path="data.txt" ("字符串")) -> (appended path=w48:path)
  n567 = Open/Create/Replace File(file path (use dialog)=w48, operation (0:open)=T8."open or create" ("操作(0:open)")) -> (refnum out=w47:refnum<file>)  [unwired: 4 in, 2 out]
  n568 = while {
    tunnel: w25 -> [w1018]
    tunnel: w26 -> [w1034]
    tunnel: w27 -> [w1033]
    tunnel: w47 -> [w1027]
    tunnel: w46 -> [w1026]
    tunnel: [w1017] -> w45
    tunnel: w24 -> [w1024]
    tunnel: [w1019] -> w21
    tunnel: w19 -> [w1007]
    tunnel: [w1016] -> w20
    tunnel: w19 -> [w1015]
    tunnel: w13 -> [w1006]
    tunnel: w12 -> [w1005]
    tunnel: [w1006] -> w11
    tunnel: [w1005] -> w10
    i -> [w1025]
    stop <- w1035 stop-if-true
    # "Mp285A控制循环"
    n569 = Dequeue Element(queue=w1033, timeout in ms (-1)=1 ("超时毫秒(-1)"), error in (no error)=w1034) -> (error out=w1036:errorcluster)  [unwired: 3 out]
    n570 = Unbundle By Name(w1036) -> ("status"=w1035:bool)
    n571 = event shown="[4] \"针尖粗对焦\": 值改变" {
      selector: _ -> [_ _ _ _ _]
      dyn-events: _ -> [_ _ _ _ _]
      timeout: 1 -> [_ _ _ _ _]
      event "自动接触": Value Change {
        n572 = event-data() -> ()  [unwired: 1 in, 6 out]
        n573 = local read "Resistance(MΩ)"() -> (w1044:dbl)
        n574 = Greater?(x=w1044, y=8.0) -> (0:w1041:bool)
        n575 = Less?(x=w1044, y=3.0) -> (x < y?=w1040:bool)
        n576 = Or(x=w1041, y=w1040) -> (x .or. y?=w1039:bool)
        n577 = local write "校准的入液阻值"(w1044) -> ()
        n578 = case shown="真" w1039 {
          frame False {
          }
          frame True {
            n579 = One Button Dialog(message="针尖异常" ("消息")) -> ()  [unwired: 1 in, 1 out]
          }
        }
        "自动接触初始" <- 0
        "针下降次数" <- 0 ("针下降次数")
      }
      event "傅里叶": Value Change {
        w1048 = u16 0 items=["傅里叶初始", "傅里叶循环", "傅里叶暂停", "傅里叶结束"] ("傅里叶状态机")
        n580 = event-data() -> ()  [unwired: 1 in, 6 out]
        n581 = local write "傅里叶状态机"(w1048) -> ()
      }
      event Timeout {
        n582 = event-data() -> ()  [unwired: 1 in, 3 out]
      }
      event "自动扫描": Value Change {
        w1049 = u16 0 items=["自动扫描初始", "自动扫描循环", "自动扫描结束"] ("自动扫描状态机")
        n583 = event-data() -> ()  [unwired: 1 in, 6 out]
        n584 = local write "自动扫描状态机"(w1049) -> ()
      }
      event "针尖粗对焦": Value Change {
        w1050 = u16 0 items=["自动对焦初始", "自动对焦循环", "自动对焦结束"] ("自动对焦状态机")
        n585 = event-data() -> ()  [unwired: 1 in, 6 out]
        n586 = local write "自动对焦状态机"(w1050) -> ()
      }
    }
    n587 = case shown="真" "自动移至工作位置" {
      tunnel: w1024 -> [w1233 w1242]
      tunnel: w1018 -> [w1234 w1239]
      tunnel: [w1234 w1236] -> w1020
      tunnel: [w1233 w1235] -> w1019
      frame False {
      }
      frame True {
        n588 = flat-sequence {
          tunnel: w1242 -> [w1245]
          tunnel: [w1243] -> w1241
          tunnel: w1241 -> [w1252]
          tunnel: [w1252] -> w1240
          tunnel: w1240 -> [w1262]
          tunnel: w1239 -> [w1261]
          tunnel: [w1262] -> w1238
          tunnel: [w1257] -> w1237
          tunnel: [w1264] -> w1236
          tunnel: [w1265] -> w1235
          tunnel: w1238 -> [w1265]
          tunnel: w1237 -> [w1264]
          frame #0 {
            n589 = call "285_GetPos.vi"("VISA资源名称"=w1245) -> ("Y"=→"Y":dbl, "X"=→"X":dbl, "VISA资源名称输出"=w1243:refnum<visa-resource-name>)  [unwired: 5 in, 3 out]
          }
          frame #1 {
            n590 = local read "Z轴坐标"() -> (w1248:string)
            n591 = Decimal String To Number(string=w1248) -> (number=w1247:i32)  [unwired: 2 in, 1 out]
            n592 = To Double Precision Float(number=w1247) -> (double precision float=w1249:dbl)
            n593 = Divide(x=w1249, y=10.0) -> (x/y=→"Z":dbl)
          }
          frame #2 {
            w1253 = 25722.32 ("y")
            w1254 = 3016.6 ("y")
            w1255 = -27641.6 ("y")
            # "等待针尖到达延时"
            # "标定"
            n594 = local read "Z"() -> (w1258:dbl)
            n595 = local read "Y"() -> (w1259:dbl)
            n596 = local read "X"() -> (w1260:dbl)
            n597 = Add(x=w1258, y=w1253) -> ()  [unwired: 1 out]
            n598 = Add(x=w1259, y=w1254) -> ()  [unwired: 1 out]
            n599 = Add(x=w1260, y=w1255) -> ()  [unwired: 1 out]
            n600 = call "285_Move.vi"("VISA resource name out"=w1261, "Abso_Z"=w1253, "Abso_Y"=w1254, "Abso_X"=w1255) -> ("VISA resource name out 2"=w1257:refnum<visa-resource-name>)  [unwired: 4 in, 3 out]
            n601 = Wait (ms)(milliseconds to wait=u32 30000 ("等待时间（毫秒）")) -> ()  [unwired: 1 out]
          }
          frame #3 {
            n602 = disable-structure shown="禁用" {
              frame Disabled {
              }
              frame Enabled {
                n603 = local write "自动扫描"(TRUE ("自动扫描")) -> ()
              }
            }
            n604 = local write "自动移至工作位置"(FALSE) -> ()
          }
        }
      }
    }
    n605 = flat-sequence {
      tunnel: [w1356] -> w1032
      tunnel: w1018 -> [w1355]
      tunnel: w1032 -> [w1440]
      tunnel: [w1441] -> w1031
      frame #0 {
        n606 = local read "Right"() -> (w1357:dbl)
        n607 = case shown="真" "针尖粗对焦" {
          tunnel: w1357 -> [_ w1360]
          tunnel: w1355 -> [w1358 w1361]
          tunnel: [w1358 w1362] -> w1356
          frame False {
          }
          frame True {
            # "爬山算法"
            # "聚焦有问题"
            n608 = flat-sequence {
              tunnel: w1360 -> [w1423]
              tunnel: [w1437] -> w1368
              tunnel: [w1436] -> w1366
              tunnel: [w1435] -> w1367
              frame #0 {
                n609 = case shown="0, 默认" "自动对焦状态机" {
                  tunnel: w1423 -> [w1424 w1431]
                  frame 0, Default {
                    n610 = flat-sequence {
                      tunnel: w1424 -> [w1428]
                      frame #0 {
                        n611 = Array Size(array="聚焦值数组") -> (size(s)=w1427:i32)
                        n612 = Delete From Array(array="聚焦值数组", length=w1427) -> (array with subset deleted=w1426:dbl[])  [unwired: 1 in, 1 out]
                        n613 = local write "聚焦值数组"(w1426) -> ()
                      }
                      frame #1 {
                        # "第一次赋值"
                        "调焦值2" <- w1428
                        "调焦值3" <- w1428
                        "调焦值4" <- w1428
                        "对焦变量" <- 1
                      }
                      frame #2 {
                        n614 = local write "自动对焦状态机"(1) -> ()
                      }
                    }
                  }
                  frame 1 {
                    n615 = flat-sequence {
                      tunnel: w1431 -> [w1434]
                      frame #0 {
                        n616 = local read "调焦值3"() -> (w1432:dbl)
                        n617 = local write "调焦值4"(w1432) -> ()
                      }
                      frame #1 {
                        n618 = local read "调焦值2"() -> (w1433:dbl)
                        n619 = local write "调焦值3"(w1433) -> ()
                      }
                      frame #2 {
                        n620 = local write "调焦值2"(w1434) -> ()
                      }
                    }
                  }
                }
              }
              frame #1 {
                n621 = local read "调焦值2"() -> (w1437:dbl)
                n622 = local read "调焦值3"() -> (w1436:dbl)
                n623 = local read "调焦值4"() -> (w1435:dbl)
              }
            }
            n624 = local read "聚焦值数组"() -> (w1364:dbl[])
            n625 = Insert Into Array(array=w1364, index=0 ("索引"), new element=w1360) -> (w1365:dbl[])
            n626 = local write "聚焦值数组"(w1365) -> ()
            n627 = Greater?(x=w1366, y=w1367) -> (0:w1374:bool)
            n628 = Greater Or Equal?(x=w1368, y=w1366) -> (x >= y?=w1371:bool)
            n629 = Boolean To (0,1)(Boolean=w1371) -> (0, 1=w1370:i16)
            n630 = Boolean To (0,1)(Boolean=w1374) -> (0, 1=w1369:i16)
            n631 = Multiply(x=i16 10, y=w1370) -> (x*y=w1372:i16)
            n632 = Add(x=w1372, y=w1369) -> (x+y=w1363:i16)
            "x+y 2" <- w1363
            n633 = case shown="1" w1363 {
              tunnel: w1361 -> [w1376 w1385 w1400 w1404]
              tunnel: [w1375 w1384 w1396 w1403] -> w1362
              frame 10 {
                # "4继续向上运动"
                n634 = flat-sequence {
                  tunnel: [w1382] -> w1375
                  tunnel: w1376 -> [w1381]
                  frame #0 {
                    n635 = local read "对焦变量"() -> (w1379:dbl)
                    n636 = Multiply(x=5.0 ("Z 2"), y=w1379) -> (x*y=w1377:dbl)
                    n637 = call "285_RelMove.vi"("VISA资源名称"=w1381, "Z 2"=w1377, "Y 2"=0.0, "X 2"=0.0) -> ("VISA resource name out 2"=w1382:refnum<visa-resource-name>)  [unwired: 2 in, 5 out]
                  }
                }
              }
              frame 0 {
                # "2向回运动"
                n638 = flat-sequence {
                  tunnel: w1385 -> [w1395]
                  tunnel: [w1394] -> w1384
                  frame #0 {
                    n639 = local read "对焦变量"() -> (w1388:dbl)
                    n640 = Multiply(x=-1.0 ("y"), y=w1388) -> (x*y=w1386:dbl)
                    n641 = local write "对焦变量"(w1386) -> ()
                  }
                  frame #1 {
                    n642 = local read "对焦变量"() -> (w1391:dbl)
                    n643 = Multiply(x=5.0, y=w1391) -> (x*y=w1389:dbl)
                    n644 = call "285_RelMove.vi"("VISA资源名称"=w1395, "Z 2"=w1389, "Y 2"=0.0, "X 2"=0.0) -> ("VISA resource name out 2"=w1394:refnum<visa-resource-name>)  [unwired: 2 in, 5 out]
                  }
                }
              }
              frame 11, Default {
                # "1往上运动"
                n645 = local read "对焦变量"() -> (w1398:dbl)
                n646 = Multiply(x=5.0 ("Z 2"), y=w1398) -> (x*y=w1397:dbl)
                n647 = call "285_RelMove.vi"("VISA资源名称"=w1400, "Z 2"=w1397, "Y 2"=0.0, "X 2"=0.0) -> ("VISA resource name out 2"=w1396:refnum<visa-resource-name>)  [unwired: 2 in, 5 out]
              }
              frame 1 {
                # "3最大值停止运动"
                n648 = local read "聚焦值数组"() -> (w1410:dbl[])
                n649 = Array Max & Min(array=w1410) -> (max value=w1409:dbl)  [unwired: 3 out]
                "最大值" <- w1409
                n650 = local read "Right"() -> (w1406:dbl)
                n651 = Subtract(x=w1409, y=15.0) -> (x-y=w1407:dbl)
                n652 = Greater?(x=w1406, y=w1407) -> (0:w1405:bool)
                n653 = case shown="真" w1405 {
                  tunnel: w1404 -> [w1415 w1421]
                  tunnel: [w1411 w1421] -> w1403
                  frame False {
                    n654 = local read "对焦变量"() -> (w1412:dbl)
                    n655 = Multiply(x=5.0 ("Z 2"), y=w1412) -> (x*y=w1414:dbl)
                    n656 = call "285_RelMove.vi"("VISA资源名称"=w1415, "Z 2"=w1414, "Y 2"=0.0, "X 2"=0.0) -> ("VISA resource name out 2"=w1411:refnum<visa-resource-name>)  [unwired: 2 in, 5 out]
                  }
                  frame True {
                    n657 = local write "自动对焦状态机"(0) -> ()
                    n658 = local write "针尖粗对焦"(FALSE ("针尖粗对焦")) -> ()
                    n659 = local write "针尖细对焦"(TRUE ("针尖细对焦")) -> ()
                  }
                }
              }
            }
          }
        }
      }
      frame #1 {
        n660 = case shown="真" "针尖细对焦" {
          tunnel: [w1442 w1445] -> w1441
          tunnel: w1440 -> [w1442 w1444]
          frame False {
          }
          frame True {
            n661 = local read "是否匹配到？"() -> (w1443:bool)
            n662 = case shown="真" w1443 {
              tunnel: [w1447 w1455] -> w1445
              tunnel: w1444 -> [w1447 w1449]
              frame False {
                n663 = disable-structure shown="禁用" {
                  frame Disabled {
                    n664 = local write "针尖自动移动"(TRUE ("针尖自动移动")) -> ()
                  }
                  frame Enabled {
                  }
                }
                n665 = local write "针尖细对焦"(FALSE ("针尖细对焦")) -> ()
              }
              frame True {
                n666 = local read "对焦变量"() -> (w1452:dbl)
                n667 = Multiply(x=2.0, y=w1452) -> (x*y=w1450:dbl)
                n668 = call "285_RelMove.vi"("VISA资源名称"=w1449, "Z 2"=w1450, "Y 2"=0.0, "X 2"=0.0) -> ("VISA resource name out 2"=w1455:refnum<visa-resource-name>)  [unwired: 2 in, 5 out]
              }
            }
          }
        }
        n669 = Wait (ms)(milliseconds to wait=u32 1000 ("等待时间（毫秒）")) -> ()  [unwired: 1 out]
      }
    }
    n670 = case shown="真" "自动扫描" {
      tunnel: w1020 -> [_ w1192]
      frame False {
      }
      frame True {
        n671 = case shown="2" "自动扫描状态机" {
          tunnel: w1192 -> [w1193 w1202 _]
          frame 0, Default {
            # "初始状态"
            n672 = flat-sequence {
              tunnel: w1193 -> [w1195]
              frame #0 {
                n673 = call "285_RelMove.vi"("VISA资源名称"=w1195, "Z 2"=0.0, "Y 2"=400.0 ("X 2"), "X 2"=0.0 ("Y 2")) -> ()  [unwired: 2 in, 6 out]
                "扫描变量" <- -1.0 ("扫描变量")
              }
              frame #1 {
                n674 = local write "自动扫描状态机"(u16 1) -> ()
                n675 = Wait (ms)(milliseconds to wait=u32 1000 ("等待时间（毫秒）")) -> ()  [unwired: 1 out]
              }
              frame #2 {
              }
            }
          }
          frame 1 {
            n676 = case shown="假" "手动暂停" {
              tunnel: w1202 -> [w1204 _]
              frame False {
                n677 = flat-sequence {
                  tunnel: [w1206] -> w1203
                  tunnel: w1204 -> [w1207]
                  tunnel: w1203 -> [w1219]
                  tunnel: [w1218] -> _
                  frame #0 {
                    n678 = for {
                      N: 7 -> [_]
                      shift-right: [w1215] -> w1206
                      shift-left: w1207 -> [w1216]
                      stop <- w1208 stop-if-true
                      n679 = local read "手动暂停"() -> (w1208:bool)
                      n680 = local read "扫描变量"() -> (w1212:dbl)
                      n681 = Multiply(x=100.0 ("X 2"), y=w1212) -> (x*y=w1210:dbl)
                      n682 = Wait (ms)(milliseconds to wait=u32 50 ("等待时间（毫秒）")) -> ()  [unwired: 1 out]
                      n683 = call "285_RelMove.vi"("VISA资源名称"=w1216, "Z 2"=0.0, "Y 2"=w1210, "X 2"=0.0 ("Y 2")) -> ("VISA resource name out 2"=w1215:refnum<visa-resource-name>)  [unwired: 2 in, 5 out]
                    }
                  }
                  frame #1 {
                    n684 = local read "手动暂停"() -> (w1217:bool)
                    n685 = case shown="假" w1217 {
                      tunnel: w1219 -> [w1227 w1228]
                      tunnel: [w1223 w1228] -> w1218
                      frame False {
                        n686 = call "285_RelMove.vi"("VISA资源名称"=w1227, "Z 2"=0.0, "Y 2"=0.0 ("X 2"), "X 2"=-100.0 ("Y 2")) -> ("VISA resource name out 2"=w1223:refnum<visa-resource-name>)  [unwired: 2 in, 5 out]
                        n687 = local read "扫描变量"() -> (w1222:dbl)
                        n688 = Multiply(x=w1222, y=-1.0) -> (x*y=w1220:dbl)
                        n689 = local write "扫描变量"(w1220) -> ()
                      }
                      frame True {
                      }
                    }
                  }
                }
              }
              frame True {
                n690 = flat-sequence {
                  frame #0 {
                    n691 = local write "自动扫描状态机"(2) -> ()
                  }
                  frame #1 {
                  }
                }
              }
            }
          }
          frame 2 {
            n692 = flat-sequence {
              frame #0 {
                n693 = local write "自动扫描状态机"(0) -> ()
              }
              frame #1 {
                w1231 = FALSE
                n694 = disable-structure shown="启用" {
                  frame Disabled {
                  }
                  frame Enabled {
                    n695 = local write "针尖粗对焦"(TRUE ("针尖粗对焦")) -> ()
                  }
                }
                n696 = local write "自动扫描"(w1231) -> ()
                n697 = local write "手动暂停"(w1231) -> ()
              }
            }
          }
        }
      }
    }
    n698 = case shown="真" "手动换物镜" {
      tunnel: w1020 -> [_ w1182]
      frame False {
      }
      frame True {
        n699 = flat-sequence {
          tunnel: w1182 -> [w1190]
          frame #0 {
            n700 = One Button Dialog(message="请手动更换40倍显微镜" ("消息")) -> ()  [unwired: 1 in, 1 out]
          }
          frame #1 {
            w1184 = u16 0 items=["傅里叶初始", "傅里叶循环", "傅里叶暂停", "傅里叶结束"] ("傅里叶状态机")
            n701 = call "285_RelMove.vi"("VISA资源名称"=w1190, "Z 2"=10.0, "Y 2"=0.0, "X 2"=0.0) -> ()  [unwired: 2 in, 6 out]
            n702 = local write "傅里叶状态机"(w1184) -> ()
            n703 = local write "手动换物镜"(FALSE) -> ()
            n704 = local write "傅里叶"(TRUE) -> ()
          }
        }
      }
    }
    n705 = case shown="真" "傅里叶" {
      tunnel: w1007 -> [_ w1091]
      tunnel: w1006 -> [_ w1090]
      tunnel: w1005 -> [_ w1089]
      frame False {
      }
      frame True {
        n706 = case shown="3" "傅里叶状态机" {
          tunnel: w1091 -> [w1093 w1120 _ _]
          tunnel: w1090 -> [_ w1118 _ _]
          tunnel: w1089 -> [_ w1117 _ _]
          frame 0, Default {
            n707 = flat-sequence {
              tunnel: w1093 -> [w1098]
              frame #0 {
                w1095 = FALSE
                n708 = VISA Flush I/O Buffer(VISA resource name=w1098) -> (VISA resource name out=w1109:refnum<visa-resource-name>, error out=w1110:errorcluster)  [unwired: 2 in]
                n709 = Number To Decimal String(number=30 ("数字")) -> (decimal integer string=w1111:string)  [unwired: 1 in]
                n710 = Concatenate Strings("C," ("字符串"), w1111, "\r") -> (w1112:string)
                n711 = VISA Write ("VISA写入")(VISA resource name=w1109, write buffer=w1112, error in (no error)=w1110) -> (VISA resource name out=w1103:refnum<visa-resource-name>, error out=w1102:errorcluster)  [unwired: 1 out]
                n712 = property class="Instr"(reference=w1103, error in=w1102) -> (reference out=w1104:refnum<visa-resource-name>, error out=w1105:errorcluster, "Serial Settings:Number of Bytes at Serial Port"=w1108:u32)
                n713 = VISA Read(VISA resource name=w1104, byte count=w1108, error in (no error)=w1105) -> (VISA resource name out=w1106:refnum<visa-resource-name>, error out=w1107:errorcluster)  [unwired: 2 out]
                n714 = VISA Flush I/O Buffer(VISA resource name=w1106, error in (no error)=w1107) -> ()  [unwired: 1 in, 2 out]
                n715 = Build Array(w1095, w1095, w1095, w1095) -> (→"傅里叶数组":bool[])
                "已发送图像" <- FALSE ("已发送图像")
                "傅里叶最大值" <- 0.0
              }
              frame #1 {
                w1113 = u16 1 items=["傅里叶初始", "傅里叶循环", "傅里叶结束"] ("傅里叶状态机")
                n716 = local write "傅里叶状态机"(w1113) -> ()
              }
            }
          }
          frame 1 {
            n717 = flat-sequence {
              tunnel: w1120 -> [w1122]
              tunnel: [w1121] -> w1119
              tunnel: w1119 -> [w1131]
              tunnel: w1118 -> [w1142]
              tunnel: w1117 -> [w1140]
              tunnel: [w1133] -> w1116
              tunnel: w1116 -> [w1154]
              tunnel: [w1156] -> w1115
              tunnel: [w1155] -> w1114
              tunnel: w1115 -> [w1167]
              tunnel: w1114 -> [w1166]
              frame #0 {
                n718 = Concatenate Strings("D" ("写入缓冲区"), "\r") -> (w1130:string)
                n719 = VISA Write ("VISA写入")(VISA resource name=w1122, write buffer=w1130) -> (VISA resource name out=w1125:refnum<visa-resource-name>, error out=w1127:errorcluster)  [unwired: 1 in, 1 out]
                n720 = property class="Instr"(reference=w1125, error in=w1127) -> (reference out=w1128:refnum<visa-resource-name>, error out=w1129:errorcluster, "Serial Settings:Number of Bytes at Serial Port"=w1126:u32)
                n721 = VISA Read(VISA resource name=w1128, byte count=w1126, error in (no error)=w1129) -> (VISA resource name out=w1121:refnum<visa-resource-name>)  [unwired: 3 out]
              }
              frame #1 {
                n722 = VISA Flush I/O Buffer(VISA resource name=w1131) -> ()  [unwired: 2 in, 2 out]
                n723 = Wait (ms)(milliseconds to wait=u32 100 ("等待时间（毫秒）")) -> ()  [unwired: 1 out]
              }
              frame #2 {
                n724 = local read "Image"() -> (w1141:T4)
                n725 = call "IMAQ ImageToArray"("Image"=w1141) -> ("Image Pixels (Float)"=w1143:sgl[][])  [unwired: 3 in, 4 out]
                n726 = call "IMAQ ArrayToComplexPlane"("Plane"=enum32{"Real", "Imaginary"}."Real", "Image"=w1142, "Image Pixels (float)"=w1143) -> ("Image Out"=w1144:T4)  [unwired: 2 in, 1 out]
                n727 = call "IMAQ FFT"("Image Dst"=w1140, "Image Src"=w1144) -> ("error out"=w1145:errorcluster, "Image Dst Out"=w1146:T4)  [unwired: 2 in]
                n728 = local read "傅里叶最大值"() -> (w1137:dbl)
                n729 = call "IMAQ ComplexPlaneToArray"("error in (no error)"=w1145, "Plane"=T13."Magnitude", "Image"=w1146) -> ("Image Pixels (float)"=w1147:sgl[][])  [unwired: 2 in, 1 out]
                n730 = Add Array Elements(numeric array=w1147) -> (sum=w1151:sgl)
                n731 = Greater?(x=w1137, y=w1151) -> (0:w1148:bool)
                n732 = Select(t=w1137, s=w1148, f=w1151) -> (s? t:f=w1134:dbl)
                n733 = local write "傅里叶最大值"(w1134) -> ()
                n734 = Multiply(x=w1134, y=0.9) -> (x*y=w1149:dbl)
                n735 = Multiply(x=w1134, y=0.98) -> (x*y=w1150:dbl)
                n736 = Less?(x=w1149, y=w1151) -> (x < y?=w1152:bool)
                n737 = Less?(x=w1151, y=w1150) -> (x < y?=w1153:bool)
                n738 = And(x=w1152, y=w1153) -> (x .and. y?=w1133:bool)
              }
              frame #3 {
                n739 = local read "傅里叶数组"() -> (w1159:bool[])
                n740 = local read "已发送图像"() -> (w1162:bool)
                n741 = Insert Into Array(array=w1159, index=0 ("索引"), new element=w1154) -> (w1158:bool[])
                n742 = And Array Elements(Boolean array=w1159) -> (logical AND=w1165:bool)
                n743 = Or Array Elements(Boolean array=w1159) -> (logical OR=w1164:bool)
                n744 = And(x=w1154, y=w1165) -> (x .and. y?=w1156:bool)
                n745 = Not Or(1:w1164, 2:w1154) -> (0:w1163:bool)
                n746 = Delete From Array(array=w1158) -> (array with subset deleted=w1157:bool[])  [unwired: 2 in, 1 out]
                n747 = Or(x=w1156, y=w1162) -> (x .or. y?=w1161:bool)
                n748 = And(x=w1162, y=w1163) -> (x .and. y?=w1155:bool)
                n749 = local write "已发送图像"(w1161) -> ()
                n750 = local write "傅里叶数组"(w1157) -> ()
              }
              frame #4 {
                n751 = case shown="真" w1166 {
                  frame False {
                  }
                  frame True {
                    w1169 = u16 2 items=["傅里叶初始", "傅里叶循环", "傅里叶结束"] ("傅里叶状态机")
                    n752 = local write "傅里叶状态机"(w1169) -> ()
                    n753 = One Button Dialog(message="没有细胞！！" ("消息")) -> ()  [unwired: 1 in, 1 out]
                  }
                }
                n754 = case shown="真" w1167 {
                  frame False {
                  }
                  frame True {
                    w1171 = u16 2 items=["傅里叶初始", "傅里叶循环", "傅里叶暂停", "傅里叶结束"] ("傅里叶状态机")
                    n755 = local write "傅里叶状态机"(w1171) -> ()
                    n756 = local write "图像网络检测"(TRUE ("升Z轴找针")) -> ()
                    n757 = local write "图像检测到"(FALSE) -> ()
                  }
                }
              }
            }
          }
          frame 2 {
            n758 = local read "图像检测到"() -> (w1175:bool)
            n759 = local read "图像网络检测"() -> (w1173:bool)
            n760 = Not(x=w1173) -> (.not. x?=w1177:bool)
            n761 = And(x=w1175, y=w1177) -> (x .and. y?=w1176:bool)
            n762 = Or(x=w1173, y=w1175) -> (x .or. y?=w1174:bool)
            n763 = case shown="真" w1176 {
              frame False {
              }
              frame True {
                w1179 = u16 3 items=["傅里叶初始", "傅里叶循环", "傅里叶暂停", "傅里叶结束"] ("傅里叶状态机")
                n764 = local write "傅里叶状态机"(w1179) -> ()
              }
            }
            n765 = case shown="假" w1174 {
              frame False {
                w1178 = u16 1 items=["傅里叶初始", "傅里叶循环", "傅里叶暂停", "傅里叶结束"] ("傅里叶状态机")
                n766 = local write "傅里叶状态机"(w1178) -> ()
              }
              frame True {
              }
            }
          }
          frame 3 {
            n767 = local write "升Z轴找针"(TRUE ("升Z轴找针")) -> ()
            n768 = local write "傅里叶"(FALSE ("傅里叶")) -> ()
          }
        }
      }
    }
    n769 = case shown="真" "针尖自动移动 2" {
      tunnel: [sgl[] [1024.0, 1024.0] ("针尖坐标") w1052] -> w1030
      frame False {
        # "图像中间坐标"
      }
      frame True {
        n770 = local read "目标坐标"() -> (w1052:i32[])
      }
    }
    n771 = local read "针尖坐标"() -> (w1011:sgl[])
    n772 = Or(x="针尖自动移动", y="针尖自动移动 2") -> (x .or. y?=w1014:bool)
    n773 = case shown="真" w1014 {
      tunnel: w1031 -> [w1304 w1327]
      tunnel: [w1304 w1314] -> w1009
      tunnel: w1030 -> [_ w1316]
      tunnel: w1011 -> [_ w1309]
      frame False {
      }
      frame True {
        # "模板针尖偏移量"
        # "PID控制针尖移动"
        # "可以直接用pid模块"
        n774 = Index Array(array=w1309, index=1 ("索引")) -> (element=w1306:sgl)
        n775 = Index Array(array=w1309, index=0 ("索引")) -> (element=w1305:sgl)
        n776 = Index Array(array=w1316, index=1 ("索引")) -> (element=w1325:sgl)
        n777 = Index Array(array=w1316, index=0 ("索引")) -> (element=w1326:sgl)
        n778 = Subtract(x=w1325, y=w1306) -> (x-y=w1321:sgl)
        n779 = Bundle("x"=w1306, "x"=w1325) -> ()  [unwired: 1 in, 1 out]
        n780 = Add(x=sgl 0.0 ("y"), y=w1305) -> (x+y=w1310:sgl)
        n781 = Subtract(x=w1326, y=w1310) -> (x-y=w1322:sgl)
        n782 = call-poly <vilib>:"PID.vi"("PID gains"="PID gains", "process variable"=w1310, "setpoint"=w1326) -> ("output"=w1312:dbl)  [unwired: 7 in, 1 out]
        n783 = call-poly <vilib>:"PID.vi"("PID gains"="PID gains 2", "process variable"=w1306, "setpoint"=w1325) -> ("output"=w1313:dbl)  [unwired: 7 in, 1 out]
        n784 = Bundle("x"=w1305, "x"=w1326) -> ()  [unwired: 1 in, 1 out]
        n785 = Square(x=w1322) -> (x^2=w1320:sgl)
        n786 = Square(x=w1321) -> (x^2=w1319:sgl)
        n787 = Add(x=w1320, y=w1319) -> (x+y=w1315:sgl)
        n788 = Greater?(x=w1315, y=15.0) -> (0:w1328:bool)
        n789 = case shown="假" w1328 {
          tunnel: w1327 -> [w1332 w1340]
          tunnel: [w1332 w1339] -> w1314
          tunnel: w1312 -> [_ w1338]
          tunnel: w1313 -> [_ w1337]
          frame False {
            n790 = local read "针尖自动移动"() -> (w1330:bool)
            n791 = case shown="真" w1330 {
              frame False {
                n792 = local write "针尖自动移动 2"(FALSE ("针尖自动移动 2")) -> ()
                n793 = local write "自动接触"(TRUE ("自动接触")) -> ()
              }
              frame True {
                n794 = local write "针尖自动移动"(FALSE ("针尖自动移动")) -> ()
                n795 = local write "手动换物镜"(TRUE ("手动换物镜")) -> ()
              }
            }
            n796 = One Button Dialog(message="针尖已移动到目标位置" ("消息")) -> ()  [unwired: 1 in, 1 out]
          }
          frame True {
            # "阈值范围需要调整，太大针尖检测不出来，太小程序会出现bug'"
            n797 = flat-sequence {
              tunnel: w1340 -> [w1347]
              tunnel: [w1346] -> w1339
              tunnel: w1338 -> [w1342]
              tunnel: w1337 -> [w1341]
              frame #0 {
                # "x位置p负号原因是设备转换后的"
                n798 = To Byte Integer(number=w1341) -> (8bit integer=w1345:i8)
                n799 = To Byte Integer(number=w1342) -> (8bit integer=w1344:i8)
                n800 = In Range and Coerce(upper limit=2.0 ("上限"), x=w1345, lower limit=-2.0 ("上限")) -> (coerced(x)=w1350:dbl)  [unwired: 1 out]
                n801 = In Range and Coerce(upper limit=2.0 ("上限"), x=w1344, lower limit=-2.0 ("上限")) -> (coerced(x)=w1343:dbl)  [unwired: 1 out]
                n802 = call "285_RelMove.vi"("VISA资源名称"=w1347, "Z 2"=0.0 ("Z"), "Y 2"=w1350, "X 2"=w1343) -> ("VISA resource name out 2"=w1346:refnum<visa-resource-name>)  [unwired: 2 in, 5 out]
              }
            }
          }
        }
      }
    }
    n803 = case shown="真" "自动接触" {
      tunnel: w1009 -> [w1456 w1470]
      tunnel: [w1456 w1466] -> w1029
      frame False {
      }
      frame True {
        # "阈值"
        n804 = local read "自动接触初始"() -> (w1458:i32)
        n805 = local read "校准的入液阻值"() -> (w1465:dbl)
        n806 = local read "阻值数组"() -> (w1476:dbl[])
        n807 = Index Array(array=w1476, index=0 ("索引")) -> (element=w1469:dbl)
        n808 = Index Array(array=w1476, index=1 ("索引")) -> (element=w1474:dbl)
        n809 = Index Array(array=w1476, index=2 ("索引")) -> (element=w1473:dbl)
        n810 = Multiply(x=1.08, y=w1465) -> (x*y=w1463:dbl)
        n811 = Greater Or Equal?(x=w1469, y=w1474) -> (x >= y?=w1472:bool)
        n812 = Greater Or Equal?(x=w1474, y=w1473) -> (x >= y?=w1471:bool)
        n813 = Greater?(x=w1469, y=w1463) -> (0:w1468:bool)
        n814 = And(x=w1472, y=w1471) -> (x .and. y?=w1467:bool)
        n815 = And(x=w1468, y=w1467) -> (x .and. y?=w1459:bool)
        n816 = Boolean To (0,1)(Boolean=w1459) -> (0, 1=w1460:i16)
        n817 = Multiply(x=i16 10, y=w1460) -> (x*y=w1461:i16)
        n818 = Add(x=w1461, y=w1458) -> (x+y=w1457:i32)
        n819 = case shown="10" w1457 {
          tunnel: w1470 -> [w1480 w1527 w1539]
          tunnel: [w1479 w1528 w1539] -> w1466
          frame 10 {
            n820 = flat-sequence {
              tunnel: w1480 -> [w1486]
              tunnel: [w1485] -> w1479
              frame #0 {
                # "向下运动"
                n821 = local read "下降/向右"() -> (w1484:bool)
                n822 = local read "针下降次数"() -> (w1483:i32)
                n823 = case shown="真" w1484 {
                  tunnel: [0.0 ("X 2") w1497] -> w1489
                  tunnel: [w1492 0.0 ("X 2")] -> w1488
                  tunnel: [0.0 ("Y 2") 0.0 ("Y 2")] -> w1487
                  frame False {
                    n824 = local read "下降步伐/um"() -> (w1490:dbl)
                    n825 = Multiply(x=w1490, y=-10.0) -> (x*y=w1492:dbl)
                  }
                  frame True {
                    n826 = local read "下降步伐/um"() -> (w1495:dbl)
                    n827 = Multiply(x=w1495, y=-10.0) -> (x*y=w1497:dbl)
                  }
                }
                n828 = Subtract(x=w1483, y=10) -> (x-y=w1482:i32)
                n829 = local write "针下降次数"(w1482) -> ()
                n830 = call "285_RelMove.vi"("VISA资源名称"=w1486, "Z 2"=w1489, "Y 2"=w1487, "X 2"=w1488) -> ("VISA resource name out 2"=w1485:refnum<visa-resource-name>)  [unwired: 2 in, 5 out]
              }
              frame #1 {
                n831 = Wait (ms)(milliseconds to wait=u32 50 ("等待时间（毫秒）")) -> ()  [unwired: 1 out]
              }
              frame #2 {
                # "阈值"
                n832 = local read "校准的入液阻值"() -> (w1513:dbl)
                n833 = local read "阻值数组"() -> (w1511:dbl[])
                n834 = Index Array(array=w1511, index=0 ("索引")) -> (element=w1508:dbl)
                n835 = Index Array(array=w1511, index=1 ("索引")) -> (element=w1507:dbl)
                n836 = Index Array(array=w1511, index=2 ("索引")) -> (element=w1505:dbl)
                n837 = Multiply(x=1.06, y=w1513) -> (x*y=w1506:dbl)
                n838 = Greater?(x=w1506, y=w1507) -> (0:w1504:bool)
                n839 = Greater?(x=w1506, y=w1508) -> (0:w1503:bool)
                n840 = Greater?(x=w1506, y=w1505) -> (0:w1502:bool)
                n841 = Compound Arithmetic op=AND ("复合运算")(w1503, w1504, w1502) -> (w1501:bool)
                n842 = case shown="真" w1501 {
                  frame False {
                    n843 = local write "自动接触"(FALSE ("自动接触")) -> ()
                    n844 = One Button Dialog(message="堵针" ("消息")) -> ()  [unwired: 1 in, 1 out]
                  }
                  frame True {
                    n845 = local write "自动接触初始"(1) -> ()
                  }
                }
              }
            }
          }
          frame 0, 1, Default {
            # "得试！！！"
            # "向下运动"
            n846 = case shown="真" "下降/向右" {
              tunnel: [0.0 ("X 2") "下降步伐/um"] -> w1525
              tunnel: [w1533 0.0 ("X 2")] -> w1524
              tunnel: [0.0 ("Y 2") 0.0 ("Y 2")] -> w1523
              frame False {
                n847 = local read "下降步伐/um"() -> (w1533:dbl)
              }
              frame True {
              }
            }
            n848 = call "285_RelMove.vi"("VISA资源名称"=w1527, "Z 2"=w1525, "Y 2"=w1523, "X 2"=w1524) -> ("VISA resource name out 2"=w1528:refnum<visa-resource-name>)  [unwired: 2 in, 5 out]
            n849 = local read "针下降次数"() -> (w1522:i32)
            n850 = Add(x=w1522, y=1) -> (x+y=w1520:i32)
            n851 = Greater?(x=w1520, y=1000) -> (0:w1519:bool)
            n852 = case shown="真" w1519 {
              frame False {
              }
              frame True {
                n853 = local write "自动接触"(FALSE ("自动接触")) -> ()
                n854 = One Button Dialog(message="自动接触失败" ("消息")) -> ()  [unwired: 1 in, 1 out]
              }
            }
            n855 = local write "针下降次数"(w1520) -> ()
          }
          frame 11 {
            n856 = local write "自动接触"(FALSE) -> ()
            n857 = local write "自动封接"(TRUE) -> ()
            n858 = One Button Dialog(message="电极已接触细胞" ("消息")) -> ()  [unwired: 1 in, 1 out]
          }
        }
      }
    }
    n859 = case shown="真" "升Z轴找针" {
      tunnel: w1015 -> [_ w1054]
      frame False {
      }
      frame True {
        n860 = local read "是否匹配到？"() -> (w1053:bool)
        n861 = case shown="假" w1053 {
          tunnel: w1054 -> [_ w1057]
          frame False {
            n862 = local write "针尖自动移动 2"(TRUE ("针尖自动移动 2")) -> ()
            n863 = local write "升Z轴找针"(FALSE ("升Z轴找针")) -> ()
          }
          frame True {
            n864 = flat-sequence {
              tunnel: w1057 -> [w1063]
              tunnel: [w1062] -> w1059
              tunnel: [w1061] -> w1058
              tunnel: w1059 -> [w1088]
              tunnel: w1058 -> [w1087]
              frame #0 {
                n865 = VISA Flush I/O Buffer(VISA resource name=w1063) -> (VISA resource name out=w1069:refnum<visa-resource-name>, error out=w1068:errorcluster)  [unwired: 2 in]
                n866 = Number To Decimal String(number=20 ("数字")) -> (decimal integer string=w1066:string)  [unwired: 1 in]
                n867 = Concatenate Strings("C," ("字符串"), w1066, "\r") -> (w1064:string)
                n868 = VISA Write ("VISA写入")(VISA resource name=w1069, write buffer=w1064, error in (no error)=w1068) -> (VISA resource name out=w1075:refnum<visa-resource-name>, error out=w1076:errorcluster)  [unwired: 1 out]
                n869 = property class="Instr"(reference=w1075, error in=w1076) -> (reference out=w1074:refnum<visa-resource-name>, error out=w1073:errorcluster, "Serial Settings:Number of Bytes at Serial Port"=w1070:u32)
                n870 = VISA Read(VISA resource name=w1074, byte count=w1070, error in (no error)=w1073) -> (VISA resource name out=w1072:refnum<visa-resource-name>, error out=w1071:errorcluster)  [unwired: 2 out]
                n871 = VISA Flush I/O Buffer(VISA resource name=w1072, error in (no error)=w1071) -> (VISA resource name out=w1062:refnum<visa-resource-name>, error out=w1061:errorcluster)  [unwired: 1 in]
              }
              frame #1 {
                n872 = Concatenate Strings("U" ("写入缓冲区"), "\r") -> (w1080:string)
                n873 = VISA Write ("VISA写入")(VISA resource name=w1088, write buffer=w1080, error in (no error)=w1087) -> (VISA resource name out=w1086:refnum<visa-resource-name>, error out=w1084:errorcluster)  [unwired: 1 out]
                n874 = property class="Instr"(reference=w1086, error in=w1084) -> (reference out=w1083:refnum<visa-resource-name>, error out=w1082:errorcluster, "Serial Settings:Number of Bytes at Serial Port"=w1085:u32)
                n875 = VISA Read(VISA resource name=w1083, byte count=w1085, error in (no error)=w1082) -> (VISA resource name out=w1078:refnum<visa-resource-name>, error out=w1077:errorcluster)  [unwired: 2 out]
                n876 = VISA Flush I/O Buffer(VISA resource name=w1078, error in (no error)=w1077) -> ()  [unwired: 1 in, 2 out]
              }
            }
          }
        }
      }
    }
    n877 = case shown="真" "保存数据" {
      tunnel: w1029 -> [w1287 w1303]
      tunnel: [w1278 w1303] -> w1016
      tunnel: w1027 -> [w1280 w1302]
      tunnel: w1026 -> [w1276 _]
      tunnel: [w1279 w1302] -> w1017
      tunnel: w1025 -> [w1274 _]
      frame True {
        w1270 = "\t"
        n878 = local read "Resistance(MΩ)"() -> (w1277:dbl)
        n879 = call "285_GetPos.vi"("VISA资源名称"=w1287) -> ("Z"=w1282:dbl, "Y"=w1284:dbl, "X"=w1286:dbl, "VISA资源名称输出"=w1278:refnum<visa-resource-name>)  [unwired: 5 in, 2 out]
        n880 = Quotient & Remainder(x=w1274, y=100) -> (x-y*floor(x/y)=w1272:i32)  [unwired: 1 out]
        n881 = Get Date/Time String(want seconds? (F)=TRUE ("需要秒？(F)")) -> (time string=w1268:string)  [unwired: 2 in, 1 out]
        n882 = Number To Fractional String(number=w1284) -> (F-format string=w1283:string)  [unwired: 3 in]
        n883 = Number To Decimal String(number=w1274) -> (decimal integer string=w1275:string)  [unwired: 1 in]
        n884 = Number To Fractional String(number=w1286) -> (F-format string=w1285:string)  [unwired: 3 in]
        n885 = Number To Fractional String(number=w1282) -> (F-format string=w1281:string)  [unwired: 3 in]
        n886 = Number To Fractional String(number=w1277) -> (F-format string=w1293:string)  [unwired: 3 in]
        n887 = Equal?(x=w1272, y=0) -> (x = y?=w1267:bool)
        n888 = case shown="真" w1267 {
          tunnel: w1276 -> [_ w1297]
          tunnel: w1275 -> [_ w1295]
          frame False {
          }
          frame True {
            n889 = Concatenate Strings("图像" ("字符串"), w1295, ".bmp" ("字符串")) -> (w1299:string)
            n890 = local read "Image"() -> (w1296:T4)
            n891 = Build Path(base path=w1297, name or relative path=w1299) -> (appended path=w1301:path)
            n892 = call-poly "IMAQ Write File 2"("File Path"=w1301, "Image"=w1296) -> ()  [unwired: 8 in, 2 out]
          }
        }
        n893 = Concatenate Strings(w1268, w1270, w1275, w1270, w1270, "X轴：" ("字符串"), w1285, w1270, "Y轴：" ("字符串"), w1283, w1270, "Z轴：" ("字符串"), w1281, w1270, "阻值：" ("字符串"), w1293, "\n") -> (w1288:string)
        n894 = Write to Text File(file (use dialog)=w1280, text=w1288) -> (refnum out=w1279:refnum<file>)  [unwired: 2 in, 2 out]
      }
      frame False {
      }
    }
  }
  n895 = call "IMAQ Dispose"("Image"=w10) -> ()  [unwired: 5 in, 1 out]
  n896 = call "IMAQ Dispose"("Image"=w11) -> ()  [unwired: 5 in, 1 out]
  n897 = call "SetDA.vi"("错误输入（无错误）"=w30, "DevIndex"=w31) -> ("错误输出"=w93:errorcluster, "DevIndex Output"=w94:i32)  [unwired: 8 in]
  n898 = call "SetDA.vi"("错误输入（无错误）"=w93, "DAVolt"=0.0, "DANum"=u8 1, "DevIndex"=w94) -> ("错误输出"=w92:errorcluster, "DevIndex Output"=w91:i32)  [unwired: 6 in]
  n899 = Build Array(w82, w82, w82, w82, w82, w82, w82, w82) -> (w80:bool[])
  n900 = call "SetDA.vi"("错误输入（无错误）"=w92, "DAVolt"=0.0, "DANum"=u8 2, "DevIndex"=w91) -> ("错误输出"=w89:errorcluster, "DevIndex Output"=w90:i32)  [unwired: 6 in]
  n901 = Boolean Array To Number(Boolean array=w80) -> (number=w81:u32)
  n902 = call "SetDA.vi"("错误输入（无错误）"=w89, "DAVolt"=0.0, "DANum"=u8 3, "DevIndex"=w90) -> ("错误输出"=w76:errorcluster, "DevIndex Output"=w77:i32)  [unwired: 6 in]
  n903 = To Unsigned Byte Integer(number=w81) -> (unsigned 8bit integer=w79:u8)
  n904 = call "SetDioOut.vi"("错误输入（无错误）"=w76, "DioOut"=w79, "DioChanSel"=u8 255, "DevIndex"=w77) -> ("错误输出"=w75:errorcluster, "DevIndex Output"=w74:i32)  [unwired: 6 in]
  n905 = call "StopRead.vi"("错误输入（无错误）"=w75, "DevIndex"=w74) -> ("错误输出"=w100:errorcluster, "DevIndex Output"=w101:i32)  [unwired: 8 in]
  n906 = call "IMAQ Dispose"("Image"=w128, "error in (no error)"=w127) -> ("error out"=w133:errorcluster)  [unwired: 4 in]
  n907 = call <vilib>:"IMAQdx Close Camera.vi"("error in"=w125, "Session In"=w132) -> ("error out"=w134:errorcluster)  [unwired: 9 in]
  n908 = call "SetSoftTrig.vi"("错误输入（无错误）"=w100, "Trig"=u8 0, "DevIndex"=w101) -> ("错误输出"=w99:errorcluster, "DevIndex Output"=w97:i32)  [unwired: 7 in]
  n909 = Release Queue(queue=w122, error in (no error)=w121) -> (error out=w72:errorcluster)  [unwired: 1 in, 2 out]
  n910 = call "ClearTrigger.vi"("错误输入（无错误）"=w99, "DevIndex"=w97) -> ("错误输出"=w98:errorcluster, "DevIndex Output"=w96:i32)  [unwired: 8 in]
  n911 = Merge Errors(w133, w134, w72) -> (→"错误输出":errorcluster)
  n912 = call "ClearBufs.vi"("错误输入（无错误）"=w98, "DevIndex"=w96) -> ("错误输出"=w102:errorcluster, "DevIndex Output"=w103:i32)  [unwired: 8 in]
  n913 = call "CloseDevice.vi"("错误输入（无错误）"=w102, "DevIndex"=w103) -> ("错误输出"=w60:errorcluster)  [unwired: 8 in, 1 out]
  n914 = Merge Errors(w61, w60) -> (→"错误输出 3":errorcluster)
  n915 = call "285_Update.vi"("VISA资源名称"=w21) -> ("VISA资源名称 2"=w22:refnum<visa-resource-name>)  [unwired: 9 in, 1 out]
  n916 = Close File(refnum=w45) -> ()  [unwired: 1 in, 2 out]
  n917 = call "285_Update.vi"("VISA资源名称"=w20) -> ("VISA资源名称 2"=w62:refnum<visa-resource-name>)  [unwired: 9 in, 1 out]
  n918 = VISA Close(VISA resource name=w22) -> ()  [unwired: 1 in, 1 out]
  n919 = VISA Close(VISA resource name=w62) -> ()  [unwired: 1 in, 1 out]
